vi "Main.vi"() -> ()   [LabVIEW 2019]
doc: "Self driving example made by ybbaek for ERP42."
uses:
  Ctrl/state.ctl
  <vilib>/userDefined/High Color/IMAQdx.ctl
  Ctrl/status.ctl
  Ctrl/system_hw.ctl
  Ctrl/joystick cfg.ctl
  Gmap/gmap_fgv-cmd.ctl
  Gmap/marker_info.ctl
  Ctrl/log_buffq.ctl
  Ctrl/error_modules.ctl
  Ctrl/agv_cmd_v.ctl
  Ctrl/cmd_common.ctl
  Ctrl/gps-databuf.ctl
  Ctrl/obstacle_info.ctl
  Ctrl/pid-in-params.ctl
  Ctrl/waypoint_buf.ctl
  Ctrl/pid-status.ctl
  Subvi/global_setting.vi
  Ctrl/pid-cfg.ctl
  Gmap/dll/GMap.NET.WindowsForms.dll
panel:
  out "State":T1
  out "Error Display":T3={"AGV"=0, "AGV Estop"=0, "Obstacle"=2, "Heading"=1, "Waypt"=2, "GNSS"=0, "VLP16"=0, "Cam"=0, "RPlidar"=0, "Joystic"=1}
  out "loop count out":T4
  out "Time info":T5={"Time_total"=2.602255344390869, "Time_run"=0.0, "Time_wait"=2.602255344390869} {"Time_total" format="%.1f"; "Time_run" format="%.1f"; "Time_wait" format="%.1f"}
  in  "ybbaek copyright":string="Made by ybbaek"
  in  "Tab_main":enum32{"Main UI", "Sub UI", "Config", "System"}(tab)
  out "point all":T6(graph)
  out "Image_color":T7(plugin-control)
  out "LiDAR Display":T8(graph)=[{"Array out"=[{"x"=0.0, "y"=0.0}, {"x"=0.7193398003386512, "y"=0.6946583704589973}, {"x"=0.0, "y"=0.0}, {"x"=-0.9271838545667873, "y"=0.37460659341591224}]}, {"Array out"=[{"x"=0.037211895365512664, "y"=0.3432387468560421}, {"x"=0.04793422512858862, "y"=0.3514966181363937}, {"x"=0.05832058142901035, "y"=0.36436205864741483}, {"x"=0.5627341150394717, "y"=3.0408693766373363}, {"x"=0.64680532100145, "y"=3.034839678916205}, {"x"=0.7366873283364822, "y"=3.05750172203851}, {"x"=0.8158698786760423, "y"=3.031635959522373}, {"x"=0.9331451610257764, "y"=3.131420821041812}, {"x"=0.004899685467144683, "y"=0.014968486307006838}, {"x"=1.049914434873501, "y"=2.9393674901148814}, {"x"=1.0224338842359812, "y"=1.9719484057312768}, {"x"=1.056603656991572, "y"=1.7959963180730734}, {"x"=1.0610931358520728, "y"=1.6950166428526934}, {"x"=1.0578713664954669, "y"=1.5944875107535377}, {"x"=1.0665021443408391, "y"=1.5125636312619686}, {"x"=1.077433024477614, "y"=1.4428578032034274}, {"x"=1.0850032011048054, "y"=1.3740064104989924}, {"x"=1.095072225331472, "y"=1.313035370356632}, {"x"=0.13957607278118947, "y"=0.14149234045339731}, {"x"=0.14291599956060283, "y"=0.13703655377158958}, {"x"=0.1465133078236048, "y"=0.1320659423567849}, {"x"=0.1386578275100177, "y"=0.09964722459859167}, {"x"=0.14122077174109132, "y"=0.09553503874940641}, {"x"=0.1444688686324124, "y"=0.09054830752736777}, {"x"=0.14738443732694032, "y"=0.08866694780932297}, {"x"=0.14995457808021992, "y"=0.08424740062923733}, {"x"=0.15169045746791707, "y"=0.08108023873407158}, {"x"=0.1550803380410649, "y"=0.07610946887916797}, {"x"=0.5644290746383124, "y"=0.24359265629927856}, {"x"=0.5639582150498643, "y"=0.2251748080442638}, {"x"=0.41414950492205704, "y"=0.14933268253404902}, {"x"=0.4146181630277808, "y"=0.13646988271215205}, {"x"=0.4184586846717039, "y"=0.12594176917459707}, {"x"=0.44769458462526207, "y"=0.12192439828522457}, {"x"=0.4515514564372801, "y"=0.10997201775620523}, {"x"=0.4606289556921582, "y"=0.0994863190491623}, {"x"=0.4600799668226086, "y"=0.08708895813194327}, {"x"=0.4048614011129938, "y"=0.06310553374168962}, {"x"=0.40636024710491037, "y"=0.05259669260358649}, {"x"=0.4111820157171695, "y"=0.04129058549797192}, {"x"=0.4536741901985323, "y"=0.03470920839929828}, {"x"=0.5839992182281244, "y"=0.000955567339076485}, {"x"=0.586069487141582, "y"=-0.014547121419821205}, {"x"=0.5882933358739553, "y"=-0.06150773094736755}, {"x"=0.5992636657008293, "y"=-0.0793933811523641}, {"x"=0.575868798189793, "y"=-0.09249697168796123}, {"x"=0.4794815805850259, "y"=-0.09211664550821055}, {"x"=0.5207405070619217, "y"=-0.1136588065434995}, {"x"=0.40395494215122685, "y"=-0.10247422706026608}, {"x"=0.37792320123187456, "y"=-0.10781026839152218}, {"x"=0.3495071946982059, "y"=-0.1103039929204306}, {"x"=0.3289166799304172, "y"=-0.11365657773992448}, {"x"=0.30733030791446936, "y"=-0.11672465179728503}, {"x"=0.3050947287304734, "y"=-0.1251090284546997}, {"x"=0.3038469355038735, "y"=-0.13379476740480148}, {"x"=0.30405676193652464, "y"=-0.27167912695066504}, {"x"=0.3099218476849613, "y"=-0.29154536238386586}, {"x"=0.3388604334873547, "y"=-0.33500127853004097}, {"x"=0.34325151630072614, "y"=-0.35700274376712055}, {"x"=0.3407582247030446, "y"=-0.37473468253849856}, {"x"=0.3258029246355666, "y"=-0.39787625814932875}, {"x"=0.3155139482560953, "y"=-0.40703310486476396}, {"x"=0.1343419152206783, "y"=-0.4670634323246042}, {"x"=0.11070702115716548, "y"=-0.43049297957865346}, {"x"=0.11046424140565235, "y"=-0.4761031546531421}, {"x"=0.09739123596280085, "y"=-0.4786932182072753}, {"x"=0.004218583737141675, "y"=-0.07688435179705115}, {"x"=0.05802099448158526, "y"=-0.4868045056276368}, {"x"=0.04608558674643472, "y"=-0.4956119260008145}, {"x"=0.01557949333511481, "y"=-0.7515885456068507}, {"x"=-0.0018576833489375396, "y"=-0.8514979735810151}, {"x"=-0.022647220319522755, "y"=-0.7616633793296085}, {"x"=-0.09417492708361101, "y"=-0.868659971225103}, {"x"=-0.11785941611955293, "y"=-0.8642506699632683}, {"x"=-0.14229004286206018, "y"=-0.8707000667292458}, {"x"=-0.1609050630122117, "y"=-0.841250147516799}, {"x"=-0.2067671415164568, "y"=-0.9523117132478806}, {"x"=-0.20605198625482285, "y"=-0.834178123340838}, {"x"=-0.2333515117149486, "y"=-0.847719077572487}, {"x"=-0.2594279084234967, "y"=-0.8518728839040539}, {"x"=-0.3389774409953587, "y"=-1.0251606493600105}, {"x"=-0.3728374985757233, "y"=-1.0348875299547278}, {"x"=-0.21982257555849657, "y"=-0.5453641309023074}, {"x"=-0.23306171365272346, "y"=-0.5352067825889877}, {"x"=-0.27818218393019845, "y"=-0.601266099612996}, {"x"=-0.2924118709245134, "y"=-0.5888985886741671}, {"x"=-0.30550719069246923, "y"=-0.5757112287728938}, {"x"=-0.285138558869652, "y"=-0.5004717796696813}, {"x"=-0.4124354308366926, "y"=-0.6129017685490489}, {"x"=-0.3722032482985255, "y"=-0.5194090314540422}, {"x"=-0.7050699279609969, "y"=-0.8482248503109743}, {"x"=-0.3534212598641885, "y"=-0.3929448600961842}, {"x"=-0.3687859639279288, "y"=-0.38861931926983306}, {"x"=-0.39927061762438265, "y"=-0.399052908649773}, {"x"=-0.7643321273706124, "y"=-0.6644237816101362}, {"x"=-0.767297911014162, "y"=-0.6311070953121213}, {"x"=-0.7686998824150671, "y"=-0.5985512119067692}, {"x"=-0.7271779246070609, "y"=-0.5341042299628113}, {"x"=-0.730511285151404, "y"=-0.5070688560407197}, {"x"=-0.7276478769936012, "y"=-0.47735063591316707}, {"x"=-0.7332296600619094, "y"=-0.45180286420683174}, {"x"=-0.7376706569933296, "y"=-0.4283118044264359}, {"x"=-0.7350246671034126, "y"=-0.4003844886474967}, {"x"=-0.7418987933431203, "y"=-0.37878117751021134}, {"x"=-0.7475662617627721, "y"=-0.35657081593147044}, {"x"=-0.5041435086062458, "y"=-0.21986205386601904}, {"x"=-0.48584433979299657, "y"=-0.19629385494993803}, {"x"=-0.4760784578208513, "y"=-0.1765201532373003}, {"x"=-0.4679334959572237, "y"=-0.15912669751255104}, {"x"=-0.46186928933121624, "y"=-0.14300003347089568}, {"x"=-0.4560366343728139, "y"=-0.12740815558635363}, {"x"=-0.4502754175244038, "y"=-0.1130491524657474}, {"x"=-0.4467093644643722, "y"=-0.09877749591803121}, {"x"=-0.44298273088963747, "y"=-0.08598175756263068}, {"x"=-0.4393424368145555, "y"=-0.07228959616603416}, {"x"=-0.4376169524302142, "y"=-0.06028652789547273}, {"x"=-0.43629870361981704, "y"=-0.048625520250862364}, {"x"=-0.43597758286292637, "y"=-0.036466385082705326}, {"x"=-0.4337740523176188, "y"=-0.025106205128448075}, {"x"=-0.43357219121954194, "y"=-0.012418433922397894}, {"x"=-0.4359989623973254, "y"=-0.0009512036877710461}, {"x"=-0.43962337625886316, "y"=0.010552229468602261}, {"x"=-0.4404266860988643, "y"=0.022479639053429236}, {"x"=-0.44495895343541736, "y"=0.0339203811543749}, {"x"=-0.45280773239569483, "y"=0.047092674405568156}, {"x"=-0.4578160839367756, "y"=0.06014562152638581}, {"x"=-0.46552826933189745, "y"=0.07321197274249847}, {"x"=-0.47641106321124965, "y"=0.08816319441766314}, {"x"=-0.4901086875913299, "y"=0.10389645974480644}, {"x"=-0.5103178534645616, "y"=0.12222213766467285}, {"x"=-0.5370139372294994, "y"=0.17400080810522456}, {"x"=-0.46408149329591586, "y"=0.1656228549453027}, {"x"=-0.4656495005595963, "y"=0.18005861581329152}, {"x"=-0.4663323638082487, "y"=0.19510093916998753}, {"x"=-0.46745010045348906, "y"=0.210111050604253}, {"x"=-0.4680972244411454, "y"=0.22531142552142344}, {"x"=-0.3747706718906415, "y"=0.1956131539304991}, {"x"=-0.36683941231682005, "y"=0.204521014986358}, {"x"=-0.3667965791811537, "y"=0.21713896932840876}, {"x"=-0.37017299397228004, "y"=0.23130975883779384}, {"x"=-0.318220561410615, "y"=0.21313065076500143}, {"x"=-0.3213045287871339, "y"=0.2276015427910756}, {"x"=-0.24212538367337458, "y"=0.227520023472707}, {"x"=-0.17947946669285567, "y"=0.18184435937264626}, {"x"=-0.16924099319043878, "y"=0.18298373896036188}, {"x"=-0.1677860822391545, "y"=0.1906930271584037}, {"x"=-0.16954711267984662, "y"=0.20105416330413897}, {"x"=-0.17052850865758717, "y"=0.2131877757635724}, {"x"=-0.17180789851886022, "y"=0.22645111725609354}, {"x"=-0.17303310157237145, "y"=0.24077332858986972}, {"x"=-0.1745382370945011, "y"=0.2558934666847587}, {"x"=-0.17570834500136337, "y"=0.27251539405487146}, {"x"=-0.148514703144379, "y"=0.24762864424362738}, {"x"=-0.13531890973055075, "y"=0.24055101884908958}, {"x"=-0.12622349307376365, "y"=0.23896169629515426}, {"x"=-0.11776445083836014, "y"=0.23962582106012587}, {"x"=-0.10315605611142512, "y"=0.2424687156883059}, {"x"=-0.09858183094858941, "y"=0.24867221920999485}, {"x"=-0.09247908731977739, "y"=0.2547324447503713}, {"x"=-0.0881002983385431, "y"=0.262352625168226}, {"x"=-0.0873557497448522, "y"=0.33892325530496537}, {"x"=-0.06613864879492504, "y"=0.32968127280083953}, {"x"=-0.06185317464036562, "y"=0.35134704678836914}, {"x"=-0.00018341309306920187, "y"=0.0012364706374559762}, {"x"=-0.042421581193537373, "y"=0.34943441365875816}, {"x"=-0.03273550342374527, "y"=0.3499723372148061}, {"x"=-0.024293544189698438, "y"=0.3501582837956332}, {"x"=-0.014938511138139295, "y"=0.3509321920043467}, {"x"=-0.004789280494373356, "y"=0.3512173476529117}, {"x"=0.0048920138106873946, "y"=0.35171598016137395}, {"x"=0.013560524982257915, "y"=0.352489254676232}, {"x"=0.02302380955838009, "y"=0.35274942125171443}, {"x"=0.03241116769680544, "y"=0.3434741856508718}, {"x"=0.04205573461848268, "y"=0.34721229483660243}, {"x"=0.051937519237767016, "y"=0.3554758171738643}, {"x"=0.68417575196985, "y"=3.054565206852931}, {"x"=0.7740347270876193, "y"=3.065281796387144}, {"x"=0.8538929235576769, "y"=3.0403668981059053}, {"x"=0.9711284589486772, "y"=3.1366035398532546}, {"x"=1.041383507715918, "y"=3.0678168870317686}, {"x"=1.0278480103439231, "y"=1.9318298398492655}, {"x"=1.040399634162634, "y"=1.8342287653764067}, {"x"=1.0503970797857973, "y"=1.7406191354737743}, {"x"=1.0601277685845496, "y"=1.655088929416164}, {"x"=1.062001244562704, "y"=1.5625040540898663}, {"x"=1.0700991338114112, "y"=1.4838996239018554}, {"x"=1.0845254893266352, "y"=1.420586859541092}, {"x"=1.0854238645260335, "y"=1.3448803280654271}, {"x"=1.0877327010534705, "y"=1.2763880957839278}, {"x"=0.14087035389941074, "y"=0.13949410701622764}, {"x"=0.14466196788817007, "y"=0.13482573028440104}, {"x"=0.14687291655966134, "y"=0.1316658987029624}, {"x"=0.14175064593549874, "y"=0.11887705572089544}, {"x"=0.2036264970682614, "y"=0.16841707808802925}, {"x"=0.13592407449410887, "y"=0.10000604218205987}, {"x"=0.14135771155859755, "y"=0.0975502941200914}, {"x"=0.14225736750876022, "y"=0.09443730136697859}, {"x"=0.1453994370555474, "y"=0.08904635705030223}, {"x"=0.14872128723328512, "y"=0.08640589519051754}, {"x"=0.1497717087020608, "y"=0.08147812757093183}, {"x"=0.1529452242949335, "y"=0.07813975214557874}, {"x"=0.15682442253056755, "y"=0.07537970879456893}, {"x"=0.5647472811675264, "y"=0.2540296654209641}, {"x"=0.5638885408067102, "y"=0.23591582407053377}, {"x"=0.5645154936678932, "y"=0.21828838702252315}, {"x"=0.4133143110507845, "y"=0.14420937133423556}, {"x"=0.4152953038207189, "y"=0.1319388992089019}, {"x"=0.42070181991580574, "y"=0.12187689986018242}, {"x"=0.41019463382308746, "y"=0.10632226898793665}, {"x"=0.4607697813923746, "y"=0.10796652747784073}, {"x"=0.4595728307656681, "y"=0.09480704468566964}, {"x"=0.4615395686039659, "y"=0.08190109347783492}, {"x"=0.4039610364961172, "y"=0.05902155108926479}, {"x"=0.4078632344447768, "y"=0.04861218456565249}, {"x"=0.4148145551337871, "y"=0.03743173585553142}, {"x"=0.4555144394149477, "y"=0.029980751899943522}, {"x"=0.4454442737995556, "y"=-0.007046200336816244}, {"x"=0.40558405794575164, "y"=-0.01837313093234705}, {"x"=0.5870349933318487, "y"=-0.06834410438272143}, {"x"=0.5825244442519296, "y"=-0.0836511915574467}, {"x"=0.4929294557879973, "y"=-0.10014764908148785}, {"x"=0.4196071385781955, "y"=-0.09844211118326883}, {"x"=0.3942699940919931, "y"=-0.10495318841607298}, {"x"=0.36809742892892505, "y"=-0.109363077937277}, {"x"=0.3385160682701253, "y"=-0.11019469825239267}, {"x"=0.3182903986529594, "y"=-0.11447394736506725}, {"x"=0.3032784647494663, "y"=-0.11889169575376882}, {"x"=0.3049481648503731, "y"=-0.12807099302492214}, {"x"=0.3046065295002057, "y"=-0.13761513247401344}, {"x"=0.3043912180306484, "y"=-0.2637300682247252}, {"x"=0.3054171367735939, "y"=-0.27986324350478725}, {"x"=0.31311274043158194, "y"=-0.30088781012102306}, {"x"=0.3523944987568351, "y"=-0.3547084961569415}, {"x"=0.3415368298179463, "y"=-0.3634613547241401}, {"x"=0.3524178717309416, "y"=-0.39485086575140443}, {"x"=0.31908555382111603, "y"=-0.39913081733019773}, {"x"=0.12997044339241726, "y"=-0.47115204164301194}, {"x"=0.10505526757844699, "y"=-0.42881889038849597}, {"x"=0.1046592082535379, "y"=-0.4763890349575047}, {"x"=0.06527164362595625, "y"=-0.4805877781824733}, {"x"=0.05278646127519131, "y"=-0.48689696241201047}, {"x"=0.3386987778362214, "y"=-3.274027395714985}, {"x"=0.025957529292859365, "y"=-0.7207827475550524}, {"x"=0.01162380532798078, "y"=-0.8524207512430099}, {"x"=-0.011422689634622552, "y"=-0.8376721224091865}, {"x"=-0.08307037095562, "y"=-0.898668772946571}, {"x"=-0.10411225420149112, "y"=-0.8634962078811257}, {"x"=-0.12842874128580306, "y"=-0.8690617402761119}, {"x"=-0.14986750133717497, "y"=-0.8595324205886313}, {"x"=-0.17043851785727526, "y"=-0.8365642677825866}, {"x"=-0.2150687033246629, "y"=-0.9373945355880031}, {"x"=-0.21778331896159028, "y"=-0.8373935684503878}, {"x"=-0.24578382552810385, "y"=-0.8553889823400642}, {"x"=-0.28307706457464193, "y"=-0.8961012431705494}, {"x"=-0.35544480560474834, "y"=-1.034118581289691}, {"x"=-0.2141042776522463, "y"=-0.5559473183594016}, {"x"=-0.22620957901224753, "y"=-0.5419333804658113}, {"x"=-0.24236435690757, "y"=-0.5403883612743524}, {"x"=-0.28505726329887, "y"=-0.5955438011939664}, {"x"=-0.29777273816175426, "y"=-0.5828392972403725}, {"x"=-0.31132675134567095, "y"=-0.5711618893943736}, {"x"=-0.29361851874449085, "y"=-0.5022163158941484}, {"x"=-0.418055248346186, "y"=-0.6054402297751684}, {"x"=-0.7024675187103798, "y"=-0.8713552362021372}, {"x"=-0.3493476679235393, "y"=-0.3992323345075954}, {"x"=-0.3598912709755358, "y"=-0.3897544394559393}, {"x"=-0.3784374459844478, "y"=-0.3897507690521831}, {"x"=-0.41910536477373445, "y"=-0.41028397874871375}, {"x"=-0.7630706703020157, "y"=-0.6467017972951926}, {"x"=-0.7653163194517437, "y"=-0.614917875558059}, {"x"=-0.771485862982975, "y"=-0.5863195060864123}, {"x"=-0.7256074092092951, "y"=-0.5196634850560259}, {"x"=-0.7225359964678987, "y"=-0.48907870921574637}, {"x"=-0.7316420792426782, "y"=-0.46610741024087005}, {"x"=-0.7351413730499343, "y"=-0.4414446869430613}, {"x"=-0.7371148283931629, "y"=-0.4151839709850541}, {"x"=-0.733924960023978, "y"=-0.3886957718496593}, {"x"=-0.743501136253052, "y"=-0.36892554857372045}, {"x"=-0.5212418238111429, "y"=-0.23617159780556485}, {"x"=-0.4960873673387058, "y"=-0.20818579194304304}, {"x"=-0.48117061967940855, "y"=-0.18636210654887417}, {"x"=-0.47138059339341626, "y"=-0.168227780619227}, {"x"=-0.46513920483608606, "y"=-0.1516940428113563}, {"x"=-0.4590349480681474, "y"=-0.13597234627700297}, {"x"=-0.45373331656080873, "y"=-0.12064960606122574}, {"x"=-0.4479402014885775, "y"=-0.10573380911691682}, {"x"=-0.44457945085334866, "y"=-0.09323183136104837}, {"x"=-0.4406259337607172, "y"=-0.07955406336257143}, {"x"=-0.438200982952092, "y"=-0.06671177587068398}, {"x"=-0.4366171481572478, "y"=-0.05445609180828143}, {"x"=-0.4354166419328846, "y"=-0.04264502231081791}, {"x"=-0.4339237471993289, "y"=-0.030580739305859018}, {"x"=-0.4335765385183767, "y"=-0.019167296273147325}, {"x"=-0.4336899858120299, "y"=-0.0072151719564631945}, {"x"=-0.43822888027642554, "y"=0.004302440199505958}, {"x"=-0.43970624941831693, "y"=0.016075267415408327}, {"x"=-0.44215144199202855, "y"=0.027406246448023953}, {"x"=-0.4482228403567289, "y"=0.039953540300533656}, {"x"=-0.45564325347687923, "y"=0.053299043715665406}, {"x"=-0.46126829400407676, "y"=0.06623866655186098}, {"x"=-0.4697270563321256, "y"=0.0800546222872615}, {"x"=-0.4827653473306562, "y"=0.0961648684120708}, {"x"=-0.49943682417100876, "y"=0.11272470298021144}, {"x"=-0.5273462266081955, "y"=0.13255195125722483}, {"x"=-0.5907054678168859, "y"=0.1638171245359714}, {"x"=-0.5561032586373484, "y"=0.17167750502882528}, {"x"=-0.4638415561984629, "y"=0.17284678401228107}, {"x"=-0.46528947420424066, "y"=0.18710412928297776}, {"x"=-0.46758216578865297, "y"=0.20300734158249711}, {"x"=-0.4675470533001976, "y"=0.21771039352842617}, {"x"=-0.46980834082055095, "y"=0.2348780223763838}, {"x"=-0.3716843976287295, "y"=0.2008904143043377}, {"x"=-0.36512371869559074, "y"=0.20908188000375139}, {"x"=-0.361088043164779, "y"=0.2203279943253483}, {"x"=-0.3366952424332568, "y"=0.2182610277232525}, {"x"=-0.320284358249612, "y"=0.22076895130573543}, {"x"=-0.3241672532540743, "y"=0.23646808329605257}, {"x"=-0.1813842335345227, "y"=0.18029925769423935}, {"x"=-0.17445776505200078, "y"=0.1825396894186601}, {"x"=-0.16770514735426642, "y"=0.18473016416082078}, {"x"=-0.16852708540716116, "y"=0.1963420076910884}, {"x"=-0.16928188551480808, "y"=0.20776824405224062}, {"x"=-0.170922566662934, "y"=0.219881163825724}, {"x"=-0.1721789491288038, "y"=0.23428609002008804}, {"x"=-0.17346253854849844, "y"=0.24873944242984602}, {"x"=-0.17501652116040026, "y"=0.26520610818929335}, {"x"=-0.17657379175860174, "y"=0.28292038820839677}, {"x"=-0.14104420185130634, "y"=0.24245985878930137}, {"x"=-0.13009106473664403, "y"=0.23944219526993626}, {"x"=-0.12093484089413561, "y"=0.23944274212828023}, {"x"=-0.11358132542809246, "y"=0.23997819174666218}, {"x"=-0.10529675589785026, "y"=0.24072838573252747}, {"x"=-0.10043881698271782, "y"=0.24684872704373445}, {"x"=-0.09473578958399388, "y"=0.2514988919894027}, {"x"=-0.09011184118675057, "y"=0.2584935561632704}, {"x"=-0.08575197566726976, "y"=0.2686458610683589}, {"x"=-0.07276691295892505, "y"=0.3364714532890245}]}, {"Array out"=[{"x"=0.037211895365512664, "y"=0.3432387468560421}, {"x"=0.04793422512858862, "y"=0.3514966181363937}, {"x"=0.05832058142901035, "y"=0.36436205864741483}, {"x"=0.004899685467144683, "y"=0.014968486307006838}, {"x"=0.13957607278118947, "y"=0.14149234045339731}, {"x"=-0.4663323638082487, "y"=0.19510093916998753}, {"x"=-0.46745010045348906, "y"=0.210111050604253}, {"x"=-0.4680972244411454, "y"=0.22531142552142344}, {"x"=-0.3747706718906415, "y"=0.1956131539304991}, {"x"=-0.36683941231682005, "y"=0.204521014986358}, {"x"=-0.3667965791811537, "y"=0.21713896932840876}, {"x"=-0.37017299397228004, "y"=0.23130975883779384}, {"x"=-0.318220561410615, "y"=0.21313065076500143}, {"x"=-0.3213045287871339, "y"=0.2276015427910756}, {"x"=-0.24212538367337458, "y"=0.227520023472707}, {"x"=-0.17947946669285567, "y"=0.18184435937264626}, {"x"=-0.16924099319043878, "y"=0.18298373896036188}, {"x"=-0.1677860822391545, "y"=0.1906930271584037}, {"x"=-0.16954711267984662, "y"=0.20105416330413897}, {"x"=-0.17052850865758717, "y"=0.2131877757635724}, {"x"=-0.17180789851886022, "y"=0.22645111725609354}, {"x"=-0.17303310157237145, "y"=0.24077332858986972}, {"x"=-0.1745382370945011, "y"=0.2558934666847587}, {"x"=-0.17570834500136337, "y"=0.27251539405487146}, {"x"=-0.148514703144379, "y"=0.24762864424362738}, {"x"=-0.13531890973055075, "y"=0.24055101884908958}, {"x"=-0.12622349307376365, "y"=0.23896169629515426}, {"x"=-0.11776445083836014, "y"=0.23962582106012587}, {"x"=-0.10315605611142512, "y"=0.2424687156883059}, {"x"=-0.09858183094858941, "y"=0.24867221920999485}, {"x"=-0.09247908731977739, "y"=0.2547324447503713}, {"x"=-0.0881002983385431, "y"=0.262352625168226}, {"x"=-0.0873557497448522, "y"=0.33892325530496537}, {"x"=-0.06613864879492504, "y"=0.32968127280083953}, {"x"=-0.06185317464036562, "y"=0.35134704678836914}, {"x"=-0.00018341309306920187, "y"=0.0012364706374559762}, {"x"=-0.042421581193537373, "y"=0.34943441365875816}, {"x"=-0.03273550342374527, "y"=0.3499723372148061}, {"x"=-0.024293544189698438, "y"=0.3501582837956332}, {"x"=-0.014938511138139295, "y"=0.3509321920043467}, {"x"=-0.004789280494373356, "y"=0.3512173476529117}, {"x"=0.0048920138106873946, "y"=0.35171598016137395}, {"x"=0.013560524982257915, "y"=0.352489254676232}, {"x"=0.02302380955838009, "y"=0.35274942125171443}, {"x"=0.03241116769680544, "y"=0.3434741856508718}, {"x"=0.04205573461848268, "y"=0.34721229483660243}, {"x"=0.051937519237767016, "y"=0.3554758171738643}, {"x"=0.14087035389941074, "y"=0.13949410701622764}, {"x"=-0.46758216578865297, "y"=0.20300734158249711}, {"x"=-0.4675470533001976, "y"=0.21771039352842617}, {"x"=-0.46980834082055095, "y"=0.2348780223763838}, {"x"=-0.3716843976287295, "y"=0.2008904143043377}, {"x"=-0.36512371869559074, "y"=0.20908188000375139}, {"x"=-0.361088043164779, "y"=0.2203279943253483}, {"x"=-0.3366952424332568, "y"=0.2182610277232525}, {"x"=-0.320284358249612, "y"=0.22076895130573543}, {"x"=-0.3241672532540743, "y"=0.23646808329605257}, {"x"=-0.1813842335345227, "y"=0.18029925769423935}, {"x"=-0.17445776505200078, "y"=0.1825396894186601}, {"x"=-0.16770514735426642, "y"=0.18473016416082078}, {"x"=-0.16852708540716116, "y"=0.1963420076910884}, {"x"=-0.16928188551480808, "y"=0.20776824405224062}, {"x"=-0.170922566662934, "y"=0.219881163825724}, {"x"=-0.1721789491288038, "y"=0.23428609002008804}, {"x"=-0.17346253854849844, "y"=0.24873944242984602}, {"x"=-0.17501652116040026, "y"=0.26520610818929335}, {"x"=-0.17657379175860174, "y"=0.28292038820839677}, {"x"=-0.14104420185130634, "y"=0.24245985878930137}, {"x"=-0.13009106473664403, "y"=0.23944219526993626}, {"x"=-0.12093484089413561, "y"=0.23944274212828023}, {"x"=-0.11358132542809246, "y"=0.23997819174666218}, {"x"=-0.10529675589785026, "y"=0.24072838573252747}, {"x"=-0.10043881698271782, "y"=0.24684872704373445}, {"x"=-0.09473578958399388, "y"=0.2514988919894027}, {"x"=-0.09011184118675057, "y"=0.2584935561632704}, {"x"=-0.08575197566726976, "y"=0.2686458610683589}, {"x"=-0.07276691295892505, "y"=0.3364714532890245}]}, {"Array out"=[]}, {"Array out"=[]}]
  in  "Tab sub":enum32{"Set ", "Info", "Map waypoint"}(tab)=enum."Info"
  in  "Speed":u16(slide)=33 scale=0.0..100.0
  in  "set state value":T1
  in  "state change":bool
  in  "full scale":bool=TRUE
  in  "ratio":dbl=10.0 format="%#_13g"
  in  "Scale_map":dbl(slide)=5.0 min=0.0 scale=5.0..100.0
  out "process_all":u8(slide) scale=0.0..100.0
  out "process_curr":dbl(slide)=nan scale=0.0..1.0
  out "stop time":dbl(slide)=2.7272372245788574 scale=0.0..5.0
  out "Pid dt":u32=100
  out "Heading":dbl
  out "Speed_control_PID":T9(graph)={"output high"=40.0, "output low"=15.0, "output"=0.0}
  out "Distance_left":dbl format="%.1f"
  out "D_gap":dbl format="%.1f"
  out "Map_Total":T10(graph)=[{"stop pt array out"=[]}, {"stop pt array out"=[]}, {"stop pt array out"=[{"X"=4530998.623923, "Y"=6178450.805513}, {"X"=4530998.538097, "Y"=6178450.804328}, {"X"=4530998.436351, "Y"=6178450.81696}, {"X"=4530998.335494, "Y"=6178450.839631}, {"X"=4530998.287734, "Y"=6178450.881083}, {"X"=4530998.369203, "Y"=6178451.026592}, {"X"=4530998.616099, "Y"=6178451.104199}, {"X"=4530998.899282, "Y"=6178451.204366}, {"X"=4530999.432829, "Y"=6178451.227778}, {"X"=4530999.994657, "Y"=6178451.1834}, {"X"=4531000.491916, "Y"=6178451.184252}, {"X"=4531000.925496, "Y"=6178451.240374}, {"X"=4531001.380332, "Y"=6178451.342912}, {"X"=4531001.869676, "Y"=6178451.447932}, {"X"=4531002.371383, "Y"=6178451.498979}, {"X"=4531002.905819, "Y"=6178451.53243}, {"X"=4531003.356208, "Y"=6178451.584774}, {"X"=4531003.754389, "Y"=6178451.628375}, {"X"=4531004.172048, "Y"=6178451.698315}, {"X"=4531004.577345, "Y"=6178451.822228}, {"X"=4531004.966722, "Y"=6178451.959958}, {"X"=4531005.304781, "Y"=6178452.098985}, {"X"=4531005.558793, "Y"=6178452.256904}, {"X"=4531005.663298, "Y"=6178452.468907}, {"X"=4531005.735073, "Y"=6178452.698506}, {"X"=4531005.808628, "Y"=6178452.948183}, {"X"=4531005.871598, "Y"=6178453.271912}, {"X"=4531005.874357, "Y"=6178453.496547}, {"X"=4531005.809877, "Y"=6178453.736296}, {"X"=4531005.695859, "Y"=6178453.997419}, {"X"=4531005.514602, "Y"=6178454.273656}, {"X"=4531005.263439, "Y"=6178454.53489}, {"X"=4531004.89372, "Y"=6178454.812535}, {"X"=4531004.439065, "Y"=6178455.099032}, {"X"=4531003.810977, "Y"=6178455.363081}, {"X"=4531003.261601, "Y"=6178455.548003}, {"X"=4531002.709556, "Y"=6178455.702809}, {"X"=4531002.017699, "Y"=6178455.827609}, {"X"=4531001.45765, "Y"=6178455.892064}, {"X"=4531000.845393, "Y"=6178455.947777}, {"X"=4531000.166788, "Y"=6178456.028643}, {"X"=4530999.390883, "Y"=6178456.172335}, {"X"=4530998.64593, "Y"=6178456.278353}, {"X"=4530997.881499, "Y"=6178456.358033}, {"X"=4530997.114399, "Y"=6178456.407596}, {"X"=4530996.505611, "Y"=6178456.308947}, {"X"=4530996.309053, "Y"=6178456.025486}, {"X"=4530996.530954, "Y"=6178455.627487}, {"X"=4530996.701536, "Y"=6178455.230783}, {"X"=4530996.904848, "Y"=6178454.816484}, {"X"=4530997.126748, "Y"=6178454.418484}, {"X"=4530997.382268, "Y"=6178454.012928}, {"X"=4530997.604168, "Y"=6178453.614928}, {"X"=4530997.677451, "Y"=6178453.281051}, {"X"=4530997.953338, "Y"=6178452.911871}, {"X"=4530998.350449, "Y"=6178452.556397}, {"X"=4530998.886482, "Y"=6178452.22089}, {"X"=4530999.254422, "Y"=6178451.923168}, {"X"=4530999.465739, "Y"=6178451.599218}, {"X"=4530999.52666, "Y"=6178451.319314}, {"X"=4530999.555832, "Y"=6178451.261562}, {"X"=4530999.57442, "Y"=6178451.277862}, {"X"=4530999.57531, "Y"=6178451.287901}, {"X"=4530999.561169, "Y"=6178451.321796}, {"X"=4530999.562948, "Y"=6178451.341874}, {"X"=4530999.582425, "Y"=6178451.368212}, {"X"=4530999.584204, "Y"=6178451.38829}, {"X"=4530999.552364, "Y"=6178451.415925}, {"X"=4530999.520524, "Y"=6178451.44356}]}]
  out "joystick":cluster{"X":dbl, "Y":dbl}[](graph)
  out "Map_Current":T11(graph)=[{"heading_curr "=[]}, {"heading_curr "=[]}, {"heading_curr "=[{"x"=0.0, "y"=0.0}, {"x"=0.0, "y"=0.0}, {"x"=0.0, "y"=0.0}, {"x"=0.0, "y"=0.0}, {"x"=0.0, "y"=0.0}, {"x"=0.0, "y"=0.0}]}, {"heading_curr "=[]}, {"heading_curr "=[{"x"=0.0, "y"=0.0}, {"x"=0.0, "y"=0.0}]}, {"heading_curr "=[{"x"=0.0, "y"=0.0}, {"x"=0.0, "y"=0.0}]}, {"heading_curr "=[{"x"=0.0, "y"=0.0}, {"x"=3.6739403974420594e-16, "y"=6.0}]}, {"heading_curr "=[{"x"=0.0, "y"=0.0}, {"x"=3.6739403974420594e-16, "y"=6.0}]}]
  in  "zoom-center":bool
  in  "GMapControl":refnum<k24>(container)
  out "Lat":dbl format="%.16f"
  out "Lon":dbl format="%.16f"
  out "Lat_DbClk":dbl format="%.16f"
  out "Lon_DbClk":dbl format="%.16f"
  in  "zoom":dbl(slide) scale=3.0..20.0
  in  "PinDropMrkr":T12(ring)=enum."red_dot" caption="Pin Drop Marker"
  in  "SetMapProvider":u16(ring)=17 items=["None", "OpenStreetMap", "OpenStreet4UMap", "OpenCycleMap", "OpenCycleLandscapeMap", "OpenCycleTransportMap", "OpenStreetMapQuest", "OpenStreetMapQuestSattelite", "OpenStreetMapQuestHybrid", "OpenSeaMapHybrid", "WikiMapiaMap", "BingMap", "BingSatelliteMap", "BingHybridMap", "YahooMap", "YahooSatelliteMap", "YahooHybridMap", "GoogleMap", "GoogleSatelliteMap", "GoogleHybridMap", "GoogleTerrainMap", "GoogleChinaMap", "GoogleChinaSatelliteMap", "GoogleChinaHybridMap", "GoogleChinaTerrainMap", "GoogleKoreaMap", "GoogleKoreaSatelliteMap", "GoogleKoreaHybridMap", "NearMap", "NearSatelliteMap", "NearHybridMap", "OviMap", "OviSatelliteMap", "OviHybridMap", "OviTerrainMap", "YandexMap", "YandexSatelliteMap", "YandexHybridMap", "LithuaniaMap", "Lithuania 2.5d Map", "LithuaniaOrtoFotoMap", "LithuaniaOrtoFotoMapOld", "LithuaniaHybridMap", "LithuaniaHybridMapOld", "LithuaniaTOP50", "LatviaMap", "MapBender, WMS demo", "TurkeyMap", "CloudMade, Demo", "SpainMap", "CzechMap", "CzechSatelliteMap", "CzechHybridMap", "CzechTuristMap", "CzechHistoryMap", "ArcGIS_Imagery_World_2D_Map", "ArcGIS_ShadedRelief_World_2D_Map", "ArcGIS_StreetMap_World_2D_Map", "ArcGIS_Topo_US_2D_Map", "ArcGIS_World_Physical_Map", "ArcGIS_World_Shaded_Relief_Map", "ArcGIS_World_Street_Map", "ArcGIS_World_Terrain_Base_Map", "ArcGIS_World_Topo_Map", "ArcGIS_DarbAE_Q2_2011_NAVTQ_Eng_V5_MapProvider"]
  out "latlong out":cluster{dbl, dbl}={530126.7583503594, 175270.68061157822} {"?" format="%.8f"; "?" format="%.8f"}
  in  "Tap_config":T13(tab)=enum."Vision"
  in  "AGV-2":enum32{"Status", "Common"}(tab)
  out "batt":dbl(slide) scale=26.0..29.0
  out "AGV velocity Chart":T14(graph)
  out "System Feedback":T15
  in  "AGV cfg":T16={"Port"="COM6", "speed limits"={"speed-limit"=0.0, "steer-limit"=0.0}, "limits"={"speed limits"={"max"=100.0, "min"=0.0}, "steer limits"={"max"=500.0, "min"=0.0}}}
  in  "Lookahead cfg":T17={"lookahead points"=64.0, "lookahead distance"=2.0} {"lookahead distance" format="%.1f"; "lookahead points" format="%#_13g"}
  in  "State machine cfg":T18
  out "Slide":cluster{dbl, dbl, dbl}(slide) scale=0.0..1.0
  out "Stop point count":u32(slide)
  in  "Tab_Lidar-config":enum32{"VLP16", "Tim571", "RPLiar A123"}(tab)
  in  "TIM571 cfg":T19 {"h range" scale=-180.0..180.0}
  in  "RPLidar cfg":T20={"port"="COM3", "dt"=4, "cicle"=28, "speed"=500, "rate"=115200} {"speed" scale=100.0..1000.0}
  out "LiDAR Display for cfg":T8(graph)=[{"Array out"=[{"x"=0.0, "y"=0.0}, {"x"=0.7193398003386512, "y"=0.6946583704589973}, {"x"=0.0, "y"=0.0}, {"x"=-0.9271838545667873, "y"=0.37460659341591224}]}, {"Array out"=[]}, {"Array out"=[]}, {"Array out"=[]}, {"Array out"=[]}]
  in  "lidat setting tab":enum32{"Range", "Limit", "Graph"}(tab)
  in  "VLP16 cfg":T21={"h range"={46, -68}, "v range"={8, -4}} {"v range" scale=-15.0..15.0; "h range" scale=-180.0..180.0}
  in  "Obstacle limit cfg":cluster{"Range":dbl, "Points":u16}={"Range"=1.0, "Points"=110} {"Points" min=10 max=5000 scale=10.0..100.0; "Range" min=0.5 max=200.0 scale=0.5..20.0}
  in  "Lidar graph scale":dbl(slide)=1.0 min=1.0 scale=1.0..10.0
  in  "decrease ratio":dbl(slide)=1.1 min=1.0 max=2.0 scale=1.0..2.0
  in  "PID cfg":T22={"PID gains"={"proportional gain (Kc)"=0.01, "integral time (Ti, min)"=0.0, "derivative time (Td, min)"=0.0}, "PID limits"={"output high"=40.0, "output low"=15.0}, "dt_pid"=100} {"PID limits"."output low" format="%.3f"; "PID limits"."output high" format="%.3f"; "PID gains"."derivative time (Td, min)" format="%.4f"; "PID gains"."integral time (Ti, min)" format="%.4f"; "PID gains"."proportional gain (Kc)" format="%.4f"}
  out "Speed_control_PID 2":T9(graph)={"output high"=40.0, "output low"=15.0, "output"=0.0}
  out "Image_binary 2":T7(plugin-control)
  in  "speed-steer_global":cluster{"speed":dbl, "steer":dbl} {"speed" scale=0.0..200.0; "steer" scale=8.0..40.0}
  in  "Record waypoint":bool
  in  "GPS cfg":T23={"Port"="COM10", "PwrPak7_heading select"="", "PwrPak7_mode select"=[]}
  out "Image_binary":T7(plugin-control)
  out "Image_gray":T7(plugin-control)
  in  "Tab vision-setting":enum32{"Port ", "Config", "camera attrib"}(tab)
  in  "camera cfg":cluster{"Port":T24, "Camera file":path}={"Port"="cam1", "Camera file"=path "C:/AGV/Config/camera/MS_LifeCam_30fps_160x120.icd"}
  in  "Vison cfg":T25 {"Threshold Range"."Upper value" scale=0.0..255.0; "Threshold Range"."Lower value" scale=0.0..255.0}
  in  "camera_attrib":cluster{"brightness":u16, "ExposureTimeAbs":dbl}={"brightness"=0, "ExposureTimeAbs"=15000.0} {"brightness" scale=0.0..10.0; "ExposureTimeAbs" scale=0.0..30000.0}
  in  "config save":bool
  in  "config load":bool
  in  "config_file-name":string="user1"
  in  "waypoint files cfg":T26={"Waypoint array"=[{"sel"=TRUE, "inv"=FALSE, "path"=path "C:/AGV/Config/waypoint/wpt_shinsung-circle_20201004-1.txt"}]}
  out "Total map cfg":T27(graph)=[{"ref waypt 0703 A \ngoal point start"=[]}, {"ref waypt 0703 A \ngoal point start"=[{"X"=4530998.623923, "Y"=6178450.805513}, {"X"=4530998.538097, "Y"=6178450.804328}, {"X"=4530998.436351, "Y"=6178450.81696}, {"X"=4530998.335494, "Y"=6178450.839631}, {"X"=4530998.287734, "Y"=6178450.881083}, {"X"=4530998.369203, "Y"=6178451.026592}, {"X"=4530998.616099, "Y"=6178451.104199}, {"X"=4530998.899282, "Y"=6178451.204366}, {"X"=4530999.432829, "Y"=6178451.227778}, {"X"=4530999.994657, "Y"=6178451.1834}, {"X"=4531000.491916, "Y"=6178451.184252}, {"X"=4531000.925496, "Y"=6178451.240374}, {"X"=4531001.380332, "Y"=6178451.342912}, {"X"=4531001.869676, "Y"=6178451.447932}, {"X"=4531002.371383, "Y"=6178451.498979}, {"X"=4531002.905819, "Y"=6178451.53243}, {"X"=4531003.356208, "Y"=6178451.584774}, {"X"=4531003.754389, "Y"=6178451.628375}, {"X"=4531004.172048, "Y"=6178451.698315}, {"X"=4531004.577345, "Y"=6178451.822228}, {"X"=4531004.966722, "Y"=6178451.959958}, {"X"=4531005.304781, "Y"=6178452.098985}, {"X"=4531005.558793, "Y"=6178452.256904}, {"X"=4531005.663298, "Y"=6178452.468907}, {"X"=4531005.735073, "Y"=6178452.698506}, {"X"=4531005.808628, "Y"=6178452.948183}, {"X"=4531005.871598, "Y"=6178453.271912}, {"X"=4531005.874357, "Y"=6178453.496547}, {"X"=4531005.809877, "Y"=6178453.736296}, {"X"=4531005.695859, "Y"=6178453.997419}, {"X"=4531005.514602, "Y"=6178454.273656}, {"X"=4531005.263439, "Y"=6178454.53489}, {"X"=4531004.89372, "Y"=6178454.812535}, {"X"=4531004.439065, "Y"=6178455.099032}, {"X"=4531003.810977, "Y"=6178455.363081}, {"X"=4531003.261601, "Y"=6178455.548003}, {"X"=4531002.709556, "Y"=6178455.702809}, {"X"=4531002.017699, "Y"=6178455.827609}, {"X"=4531001.45765, "Y"=6178455.892064}, {"X"=4531000.845393, "Y"=6178455.947777}, {"X"=4531000.166788, "Y"=6178456.028643}, {"X"=4530999.390883, "Y"=6178456.172335}, {"X"=4530998.64593, "Y"=6178456.278353}, {"X"=4530997.881499, "Y"=6178456.358033}, {"X"=4530997.114399, "Y"=6178456.407596}, {"X"=4530996.505611, "Y"=6178456.308947}, {"X"=4530996.309053, "Y"=6178456.025486}, {"X"=4530996.530954, "Y"=6178455.627487}, {"X"=4530996.701536, "Y"=6178455.230783}, {"X"=4530996.904848, "Y"=6178454.816484}, {"X"=4530997.126748, "Y"=6178454.418484}, {"X"=4530997.382268, "Y"=6178454.012928}, {"X"=4530997.604168, "Y"=6178453.614928}, {"X"=4530997.677451, "Y"=6178453.281051}, {"X"=4530997.953338, "Y"=6178452.911871}, {"X"=4530998.350449, "Y"=6178452.556397}, {"X"=4530998.886482, "Y"=6178452.22089}, {"X"=4530999.254422, "Y"=6178451.923168}, {"X"=4530999.465739, "Y"=6178451.599218}, {"X"=4530999.52666, "Y"=6178451.319314}, {"X"=4530999.555832, "Y"=6178451.261562}, {"X"=4530999.57442, "Y"=6178451.277862}, {"X"=4530999.57531, "Y"=6178451.287901}, {"X"=4530999.561169, "Y"=6178451.321796}, {"X"=4530999.562948, "Y"=6178451.341874}, {"X"=4530999.582425, "Y"=6178451.368212}, {"X"=4530999.584204, "Y"=6178451.38829}, {"X"=4530999.552364, "Y"=6178451.415925}, {"X"=4530999.520524, "Y"=6178451.44356}]}]
  in  "test waypoint":bool
  in  "stop points edit":bool
  in  "stop point config":cluster{"distance":dbl, "time":dbl}={"distance"=1.0, "time"=5.0}
  in  "Joystick cfg":T28={"Type"=enum."Logitech F710", "steer limit"={"min"=10.0, "max"=42.0, "scale"=0.0, "offset"=0.0}, "speed limit"={"min"=10.0, "max"=42.0, "pwm max"=0.0}, "ID"=0, "joystick max"=0.0}
  out "LiDAR img":T7(plugin-control)
  in  "Joystick\ncontrol":bool
  in  "HW info":T29={"AGV"=enum."Ycar", "Lidar 1"=enum."RPLidar A2", "Lidar 2"=enum."none", "GPS"=enum."none", "Camera"=enum."MS LifeCam", "Joystick"=enum."joystick"}
  in  "Steer":i16(slide) scale=-2000.0..2000.0
  in  "use event":bool
  in  "pause-resume":bool
  in  "Checking":bool
  in  "start-stop":bool
  in  "close":bool
  in  "System status":string="\r\n00:38:31.5 - System start \r\n00:38:31.5 - UDP start \r\n00:38:31.6 - Logging loop finish \r\n00:38:31.6 - Jostick fail ### \r\n00:38:31.6 - UDP finish \r\n00:38:35.1 - VLP16 loop finish \r\n00:38:35.2 - F9P loop finish \r\n00:38:35.2 - Camera loop finish \r\n00:38:35.2 - Scout finish \r\n00:38:35.2 - Tim571 hw finish \r\n00:38:35.2 - RPLidar loop finish \r\n00:38:35.2 - GPS  finish \r\n00:38:35.2 - Producer fihish \r\n00:38:35.3 - Vision loop finish \r\n00:38:35.3 - Display Lidar finish \r\n00:38:35.3 - Timer loop finish \r\n00:38:35.5 - TCP loop finish \r\n00:38:36.5 - State loop finish \r\n00:38:36.6 - Shut down "
  # "System status"
  # "Set-Info"
  # "Process"
  # "<Xbox>\njoy max: 32767\nsteer min 10 / scale 16\nsteer max 42 / offset 26\nspeed min 10 / pwm max 255\nspeed max 200"
  # "AGV"
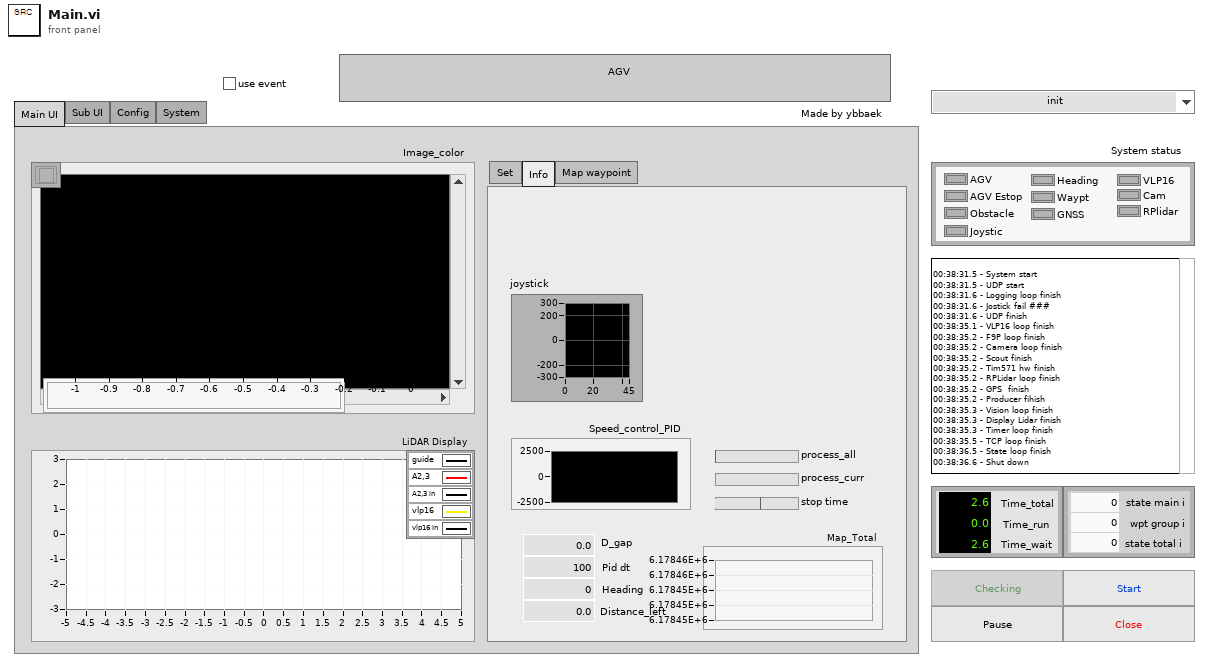
[diagram p1: front panel]
types:
  T1 = typedef "state.ctl" = enum16{"init", "Test circular track", "start point", "start heading adjust", "wait before start", "stop point check", "stop point start", "end point", "entering ending point", "move", "move heading adjust"}
  T2 = typedef "status.ctl" = u16
  T3 = cluster{"AGV":T2, "AGV Estop":T2, "Obstacle":T2, "Heading":T2, "Waypt":T2, "GNSS":T2, "VLP16":T2, "Cam":T2, "RPlidar":T2, "Joystic":T2}
  T4 = cluster{"wpt group i":i32, "state total i":i32, "state main i":i32}
  T5 = cluster{"Time_total":dbl, "Time_run":dbl, "Time_wait":dbl}
  T6 = cluster{"Points-2":cluster{"X":sgl, "Y":sgl}[]}[]
  T7 = typedef "IMAQ Image.ctl" = refnum<image>
  T8 = cluster{"Array out":cluster{"x":dbl, "y":dbl}[]}[]
  T9 = cluster{"output high":dbl, "output low":dbl, "output":dbl}
  T10 = cluster{"stop pt array out":cluster{"X":dbl, "Y":dbl}[]}[]
  T11 = cluster{"heading_curr ":cluster{"x":dbl, "y":dbl}[]}[]
  T12 = enum16{"none", "arrow", "blue", "blue_small", "blue_dot", "blue_pushpin", "brown_small", "gray_small", "green", "green_small", "green_dot", "green_pushpin", "green_big_go", "yellow", "yellow_small", "yellow_dot", "yellow_big_pause", "yellow_pushpin", "lightblue", "lightblue_dot", "lightblue_pushpin", "orange", "orange_small", "orange_dot", "pink", "pink_dot", "pink_pushpin", "purple", "purple_small", "purple_dot", "purple_pushpin", "red", "red_small", "red_dot", "red_pushpin", "red_big_stop", "black_small", "white_small"}
  T13 = enum32{"AGV", "LIDAR", "PID", "GNSS", "Vision", "File", "Waypoint", "Joystick", "Etc"}
  T14 = cluster{"Linear Velocity (m/s)":dbl, "Angular Velocity (rad/s)":dbl, "Battery Voltage":dbl}
  T15 = cluster{"state":string, "Mode":u8, "Battery V":dbl, "error High":u8, "error Low":u8}
  T16 = cluster{"Port":refnum<visa-resource-name>, "speed limits":cluster{"speed-limit":dbl, "steer-limit":dbl}, "limits":cluster{"speed limits":cluster{"max":dbl, "min":dbl}, "steer limits":cluster{"max":dbl, "min":dbl}}}
  T17 = cluster{"lookahead points":dbl, "lookahead distance":dbl}
  T18 = cluster{" turn steer speed":dbl, "move speed":dbl, "slow down factor":dbl, "adjust angle margin":dbl}
  T19 = cluster{"TIM571 IP":string, "h range":cluster{i16, i16}}
  T20 = cluster{"port":refnum<visa-resource-name>, "dt":u32, "cicle":u8, "speed":u16, "rate":u32}
  T21 = cluster{"h range":cluster{i16, i16}, "v range":cluster{i8, i8}}
  T22 = cluster{"PID gains":cluster{"proportional gain (Kc)":dbl, "integral time (Ti, min)":dbl, "derivative time (Td, min)":dbl}, "PID limits":cluster{"output high":dbl, "output low":dbl}, "dt_pid":u32}
  T23 = cluster{"Port":refnum<visa-resource-name>, "PwrPak7_heading select":string, "PwrPak7_mode select":string[]}
  T24 = typedef "IMAQdx.ctl" = refnum<k21>
  T25 = cluster{"Clamp Settings":cluster{"Contrast":i32, "Filter width":i32, "Steepness":i32, "Subsampling Ratio":u32, "Show Search Area":bool, "Show Search Lines":bool, "Show Edges Found":bool, "Show Result":bool}, "Threshold Range":cluster{"Lower value":sgl, "Upper value":sgl}, "N of Erosion 1":i32, "N of Erosion 2":i32}
  T26 = cluster{"Waypoint array":cluster{"sel":bool, "inv":bool, "path":path}[]}
  T27 = cluster{"ref waypt 0703 A \ngoal point start":cluster{"X":dbl, "Y":dbl}[]}[]
  T28 = typedef "joystick cfg.ctl" = cluster{"Type":enum16{"Logitech F710", "Xbox"}, "steer limit":cluster{"min":dbl, "max":dbl, "scale":dbl, "offset":dbl}, "speed limit":cluster{"min":dbl, "max":dbl, "pwm max":dbl}, "ID":i32, "joystick max":dbl}
  T29 = typedef "system_hw.ctl" = cluster{"AGV":enum16{"none", "ERP42", "ERP42mini", "Scout", "Ycar"}, "Lidar 1":enum16{"none", "VLP16", "TIM571", "RPLidar A2", "RPLidar A3"}, "Lidar 2":enum16{"none", "VLP16", "TIM571", "RPLidar A2", "RPLidar A3"}, "GPS":enum16{"none", "F9P", "M8P", "PwrPak7", "19X HVS"}, "Camera":enum16{"none", "C920", "C922", "GT1290C", "MS LifeCam"}, "Joystick":enum16{"none", "joystick"}}
  T30 = typedef "marker_info.ctl" = cluster{"arrLatLngActv":dbl[], "type":i32}
  T31 = typedef "gmap_fgv-cmd.ctl" = enum16{"marker type change", "save_image", "coll of points", "zoom n center markers", "add overlay reference", "read", "zoom", "set position by keyword", "set map provider", "map provider update", "create", "add marker", "clear marker", "close"}
  T32 = enum16{"Config Save", "Config Load", "LastRUN Save", "LastRUN Load"}
  T33 = cluster{"Name":string, "Color":u32, "Style":u8, "Point Style":u8, "Name Visible":bool, "Allow Drag":bool, "Annotation Mode":u32, "Plot":i32, "Index":i32, "Position":cluster{"X":dbl, "Y":dbl}, "X Scale":u32, "Y Scale":u32, "Show Arrow":bool, "Lock Name":bool, "Plot Area":i32, "Label Offset":cluster{"X":dbl, "Y":dbl}}
  T34 = enum8{"Enabled", "Disabled", "Disabled and Grayed Out"}
  T35 = typedef "error_modules.ctl" = enum16{"init", "read", "TIM571 error in", "VLP16 error in", "PwrPak7 error in"}
  T36 = typedef "log_buffq.ctl" = enum16{"create", "write", "read", "close"}
  T37 = typedef "agv_cmd_v.ctl" = enum16{"write limit", "init stop", "write", "read"}
  T38 = typedef "cmd_common.ctl" = enum16{"read", "write"}
  T39 = cluster{"VLP16 cfg":refnum<vi>, "TIM571 cfg":refnum<vi>, "PID cfg":refnum<vi>, "AGV cfg":refnum<vi>, "GPS cfg":refnum<vi>, "camera cfg":refnum<vi>, "ybbaek copyright":refnum<vi>, "Obstacle limit cfg":refnum<vi>, "State machine cfg":refnum<vi>, "Lookahead cfg":refnum<vi>, "waypoint files cfg":refnum<vi>, "Vison cfg":refnum<vi>, "RPLidar cfg":refnum<vi>, "point all":refnum<vi>, "HW info":refnum<vi>, "Joystick cfg":refnum<vi>}
  T40 = cluster{"VLP16 cfg":cluster{"h range":cluster{i16, i16}, "v range":cluster{i8, i8}}, "TIM571 cfg":cluster{"IP":string, "h range":cluster{i16, i16}}, "AGV cfg":cluster{"Port":refnum<visa-resource-name>, "speed limits":cluster{"limit_linear-v":dbl, "limit_angular-v":dbl}, "limits":cluster{"speed limits":cluster{"max":dbl, "min":dbl}, "steer limits":cluster{"max":dbl, "min":dbl}}}, "GPS cfg":cluster{"PwrPak7 Port":refnum<visa-resource-name>, "heading select":string, "mode select":string[]}, "PID cfg":cluster{"PID gains":cluster{"proportional gain (Kc)":dbl, "integral time (Ti, min)":dbl, "derivative time (Td, min)":dbl}, "PID limits":cluster{"output high":dbl, "output low":dbl}, "dt pid":u32}, "Lookahead cfg":cluster{"lookahead pts n":dbl, "lookahead distance":dbl}, "Obstacle limit range":cluster{"RL range":dbl, "Point limit":u16}, "State machine parameter":cluster{"angle adjust limit":dbl}, "waypoint group":cluster{"Waypoint array":cluster{"sel":bool, "inv":bool, "path":path}[]}, "State machine cfg":cluster{" turn angular speed":dbl, "move linear speed":dbl, "decrease factor linear speed":dbl, "adjust angle margin":dbl}, "camera cfg":cluster{"Port":T24, "Camera file":path}, "ROI-clamp":cluster{"Global Rectangle":i32[], "Contours":cluster{"Contour Type":u32, "ROI Type":u32, "Points":i32[]}[]}, "x-center":dbl, "Image Size":cluster{"x":i32, "y":i32}, "Angle deg":sgl, "Vison cfg":cluster{"Clamp Settings":cluster{"Contrast":i32, "Filter width":i32, "Steepness":i32, "Subsampling Ratio":u32, "Show Search Area":bool, "Show Search Lines":bool, "Show Edges Found":bool, "Show Result":bool}, "Range":cluster{"Lower value":sgl, "Upper value":sgl}, "N of Erosion 1":i32, "N of Erosion 2":i32}, "RPLidar cfg":cluster{"port":refnum<visa-resource-name>, "dt":u32, "update":u8, "speed":u16, "rate ":u32}, "HW info":T29, "Joystick cfg":T28}
  T41 = cluster{"Name":string, "Color":u32, "Style":u8, "Point Style":u8, "Name Visible":bool, "Allow Drag":bool, "Annotation Mode":u32, "Plot":i32, "Index":i32, "Position":cluster{"X":dbl, "Y":dbl}, "X Scale":u32, "Y Scale":u32, "Show Arrow":bool, "Lock Name":bool, "Plot Area":i32, "Label Offset":cluster{"X":dbl, "Y":dbl}}[]
  T42 = cluster{"AGV":T2, "AGV Estop":T2, "Obstacle":T2, "Heading":T2, "Waypt":T2, "GNSS":T2, "VLP16":T2, "Cam":T2, "RPLidar":T2, "Joystick":T2}
  T43 = cluster{"Global Rectangle":i32[], "Contours":cluster{"Contour Type":u32, "ROI Type":u32, "Points":i32[]}[]}
  T44 = cluster{"Lat":refnum<vi>, "Lon":refnum<vi>, "Lat_DbClk":refnum<vi>, "Lon_DbClk":refnum<vi>, "zoom":refnum<vi>, "PinDropMrkr":refnum<vi>}
  T45 = typedef "gmap_info.ctl" = cluster{"Zoon_info":cluster{"MaxZoom":dbl, "MinZoom":dbl, "Zoom":dbl}, "arrOverlayNames":string[], "MapProvider":string}
  T46 = typedef "gps-databuf.ctl" = enum16{"read", "write"}
  T47 = typedef "obstacle_info.ctl" = enum16{"init", "read", "obstacle status in", "write limit", "inrange pt-n"}
  T48 = typedef "pid-in-params.ctl" = enum16{"read", "write"}
  T49 = typedef "waypoint_buf.ctl" = enum16{"clear", "write", "read"}
  T50 = typedef "pid-status.ctl" = enum16{"read", "wirte pid dt", "wirte pid output"}
  T51 = typedef "pid-cfg.ctl" = enum16{"read", "write pid gain", "write pid limit", "pid dt"}
  T52 = cluster{"rawdata":string, "GPS Data":cluster{"Latitude":cluster{"Valid?":bool, "Latitude (Deg)":dbl}, "Longitude":cluster{"Valid?":bool, "Longitude (Deg)":dbl}, "Height":cluster{"Valid?":bool, "Height (m)":dbl}, "Undulation":cluster{"Valid?":bool, "Undulation(m)":dbl}, "North Vel":cluster{"Valid?":bool, "North Vel (m/s)":dbl}, "East Vel":cluster{"Valid?":bool, "East Vel (m/s)":dbl}, "Up Vel":cluster{"Valid?":bool, "Up Vel (m/s)":dbl}, "Roll":cluster{"Valid?":bool, "Roll (degrees)":dbl}, "Pitch":cluster{"Valid?":bool, "Pitch (degrees)":dbl}, "Azimuth":cluster{"Valid?":bool, "Azimuth (degrees)":dbl}, "Lat deviation":cluster{"Valid?":bool, "Lat deviation (m)":dbl}, "Long deviation":cluster{"Valid?":bool, "Long deviation (m)":dbl}, "Height deviation":cluster{"Valid?":bool, "Height deviation (m)":dbl}, "North vel deviation":cluster{"Valid?":bool, "North vel deviation (m/s)":dbl}, "East vel deviation":cluster{"Valid?":bool, "East vel deviation (m/s)":dbl}, "Up vel deviation":cluster{"Valid?":bool, "Up vel deviation (m/s)":dbl}, "Roll deviation":cluster{"Valid?":bool, "Roll deviation (degrees)":dbl}, "Pitch deviation":cluster{"Valid?":bool, "Pitch deviation (degrees)":dbl}, "Azimuth deviation":cluster{"Valid?":bool, "Azimuth deviation (degrees)":dbl}, "Ext sol status":cluster{"Valid?":bool, "Ext sol status":dbl}}, "Heading":dbl, "utm-1":cluster{"XN":dbl, "YE":dbl}}
  T53 = cluster{"total time":dbl, "run time":dbl, "wait time":dbl}
  T54 = cluster{"deg_agv-lookahead":dbl, "deg_waypoint":dbl, "deg_gap":dbl, "deg_target":dbl, "pid output":dbl, "distance-gap_out":dbl}
  T55 = cluster{"lookahead pt n":dbl, "lookahead distance":dbl}
  T56 = cluster{"System Feedback":cluster{"system state":string, "Control Mode":u8, "Battery Voltage":dbl, "error code High":u8, "error code Low":u8}, "Motion Feedback":cluster{"Linear Velocity (m/s)":dbl, "Angular Velocity (rad/s)":dbl}}
  T57 = cluster{"system state":string, "Control Mode":u8, "Battery Voltage":dbl, "error code High":u8, "error code Low":u8}
  T58 = cluster{"Linear Velocity (m/s)":dbl, "Angular Velocity (rad/s)":dbl}
  T59 = cluster{"start point":cluster{"x":dbl, "y":dbl}, "stop point":cluster{"x":dbl, "y":dbl}}
  T60 = cluster{"progress_curr":dbl, "progress_all":dbl, "distance_left":dbl, "distance_all":dbl}
  T61 = cluster{"output high":dbl, "output low":dbl, "pid output":dbl}
  T62 = cluster{"total time":dbl, "run time":dbl, "pause time":dbl}
  T63 = typedef "mapinfo.ctl" = cluster{"GmapDotNet":refnum<k24>, "mapprovider_info":cluster{"index":i32, "dotnetrefs":refnum<k24>, "Name":string}[]}
  T64 = cluster{"index":i32, "dotnetrefs":refnum<k24>, "Name":string}[]
  T65 = cluster{"index":i32, "dotnetrefs":refnum<k24>, "Name":string}
  T66 = typedef "data.ctl" = cluster{"Drive_value":cluster{"F/B":enum16{"Go", "N", "Back"}, "Speed":u16, "Steer":i16, "A/M":enum16{"Brake", "Auto", "Manual"}, "Brake":u8}}
  T67 = enum16{"none", "ERP42", "ERP42mini", "Scout", "Ycar"}
  T68 = enum16{"none", "VLP16", "TIM571", "RPLidar A2", "RPLidar A3"}
  T69 = enum16{"none", "F9P", "M8P", "PwrPak7", "19X HVS"}
  T70 = enum16{"none", "C920", "C922", "GT1290C", "MS LifeCam"}
  T71 = cluster{"latlong out":dbl[], "PinDropMrkr":enum16{"none", "arrow", "blue", "blue_small", "blue_dot", "blue_pushpin", "brown_small", "gray_small", "green", "green_small", "green_dot", "green_pushpin", "green_big_go", "yellow", "yellow_small", "yellow_dot", "yellow_big_pause", "yellow_pushpin", "lightblue", "lightblue_dot", "lightblue_pushpin", "orange", "orange_small", "orange_dot", "pink", "pink_dot", "pink_pushpin", "purple", "purple_small", "purple_dot", "purple_pushpin", "red", "red_small", "red_dot", "red_pushpin", "red_big_stop", "black_small", "white_small"}}
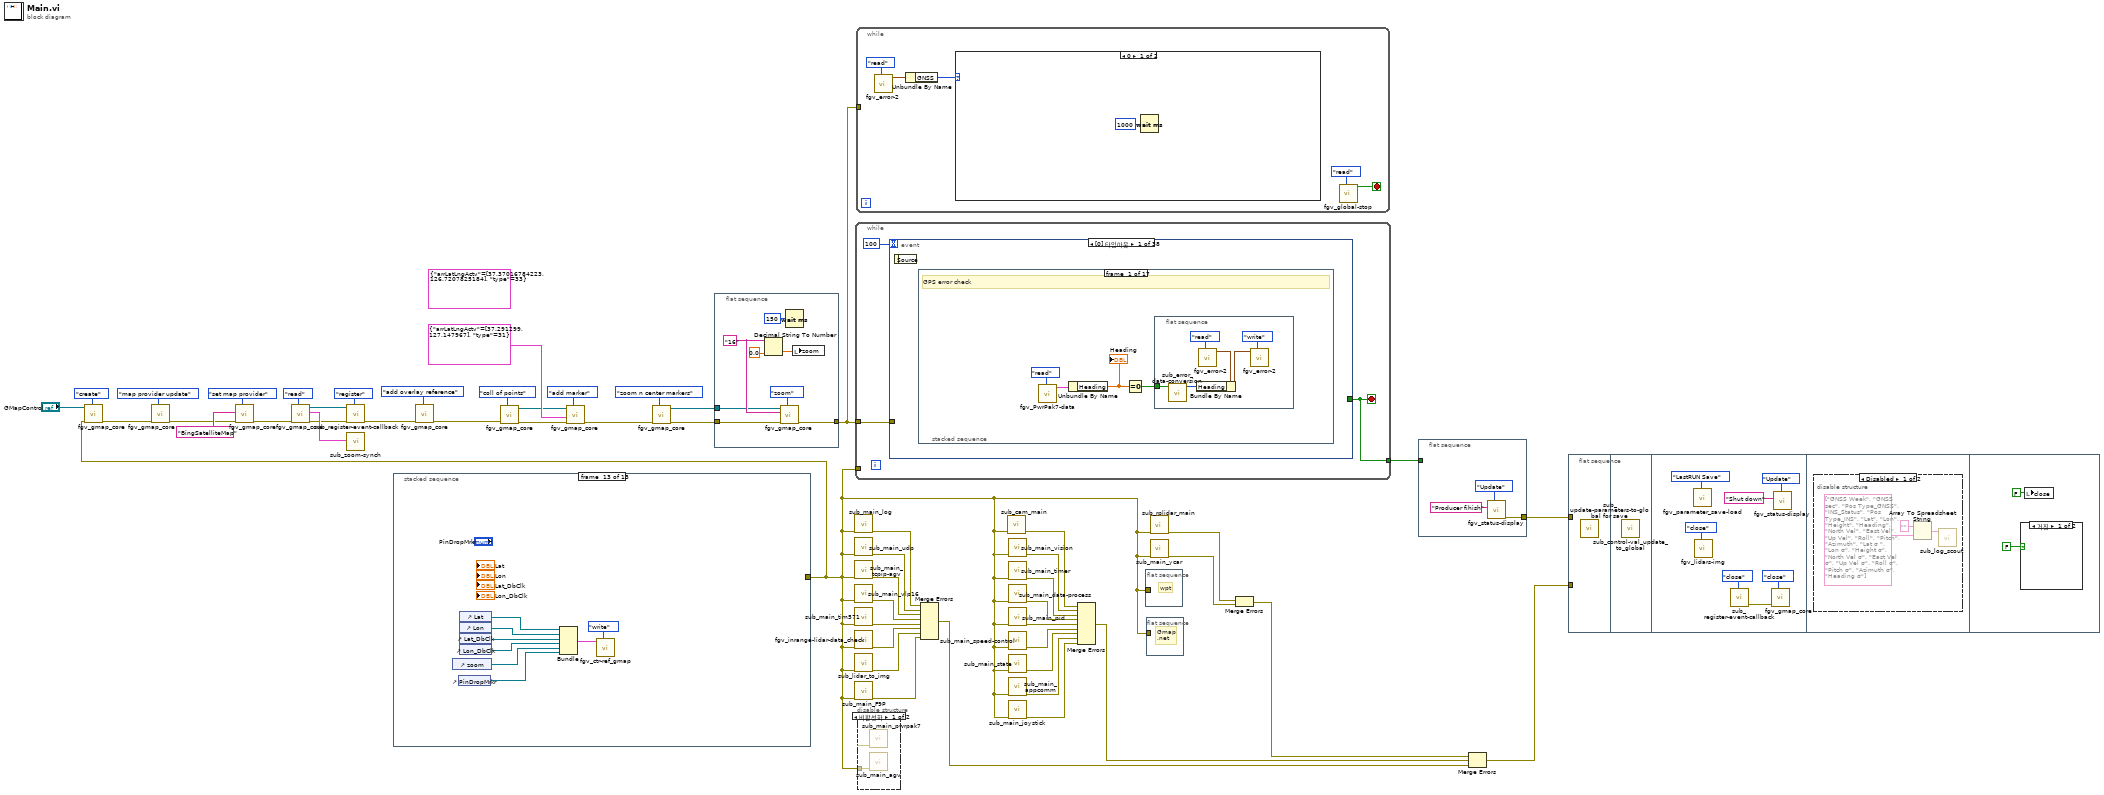
[diagram p0: block diagram]
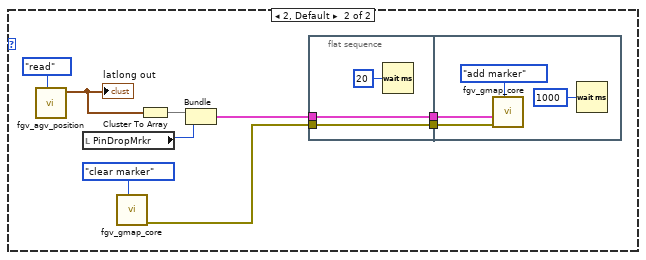
[diagram p2: hidden frame]
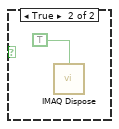
[diagram p5: hidden frame]
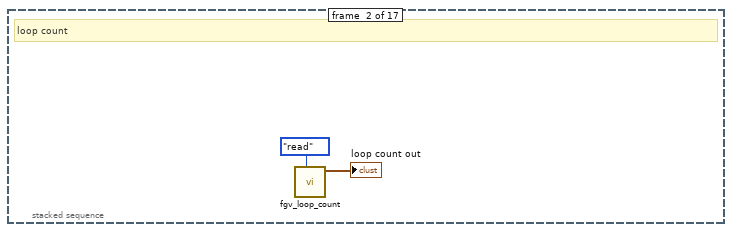
[diagram p6: hidden frame]
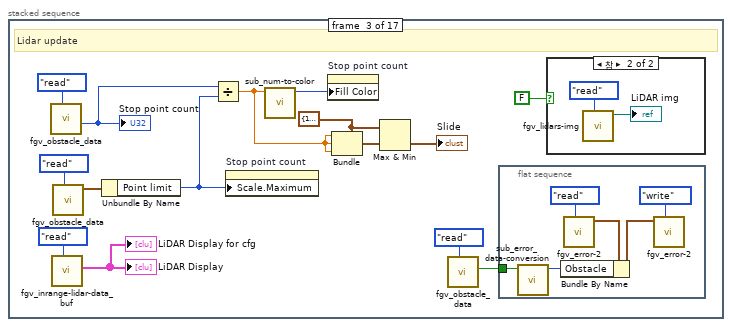
[diagram p7: hidden frame]
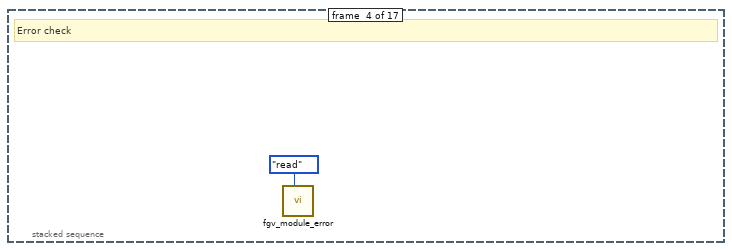
[diagram p9: hidden frame]
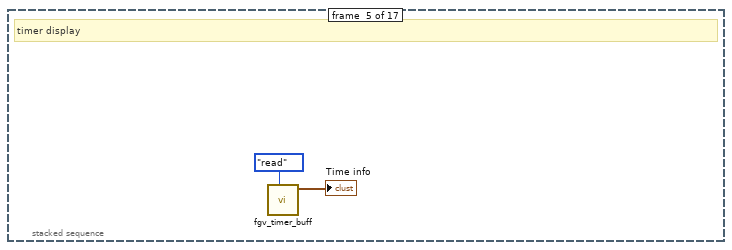
[diagram p10: hidden frame]
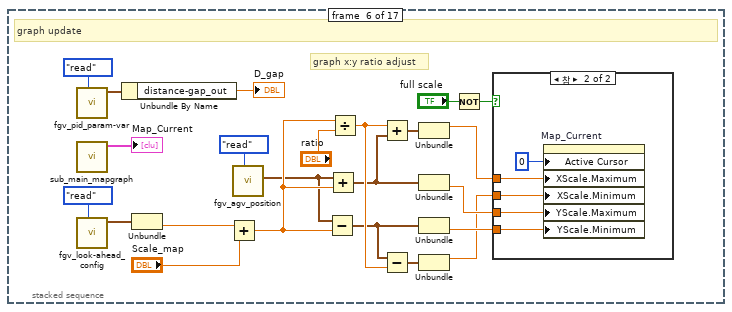
[diagram p11: hidden frame]
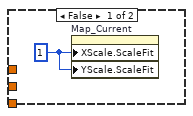
[diagram p12: hidden frame]
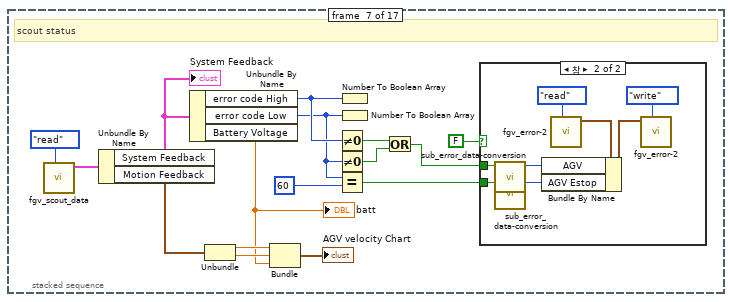
[diagram p13: hidden frame]
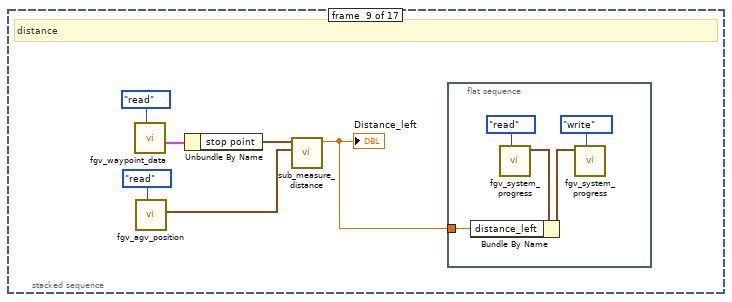
[diagram p16: hidden frame]
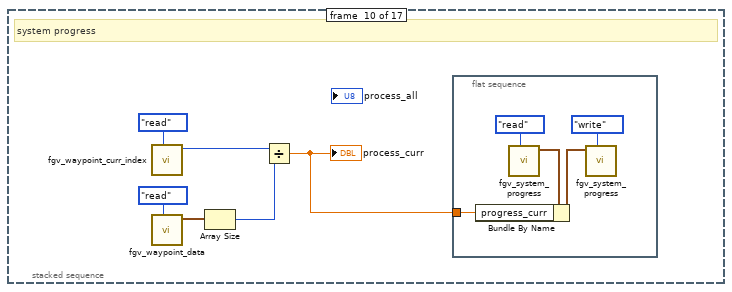
[diagram p17: hidden frame]
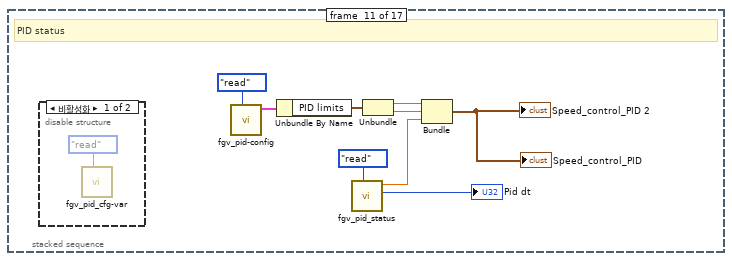
[diagram p18: hidden frame]
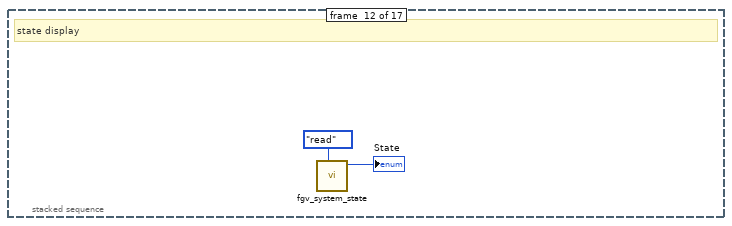
[diagram p20: hidden frame]
diagram:
  (unwired) T30 {"arrLatLngActv"=[37.37016784223, 126.7207825184], "type"=33} ("marker_info")
  n1 = stacked-sequence {
    tunnel: [_ _ _ _ w97 _ _ _ _ _ _ _ _] -> w1
    frame #0 {
      # "conrol ref - Parameter loading from file"
      n2 = control-ref of="GMapControl"() -> ()  [unwired: 1 out]
      n3 = control-ref of="point all"() -> (w58:refnum<vi>)
      n4 = control-ref of="VLP16 cfg"() -> (w63:refnum<vi>)
      n5 = control-ref of="TIM571 cfg"() -> (w71:refnum<vi>)
      n6 = control-ref of="PID cfg"() -> (w70:refnum<vi>)
      n7 = control-ref of="AGV cfg"() -> (w69:refnum<vi>)
      n8 = control-ref of="GPS cfg"() -> (w68:refnum<vi>)
      n9 = control-ref of="camera cfg"() -> (w62:refnum<vi>)
      n10 = control-ref of="Obstacle limit cfg"() -> (w67:refnum<vi>)
      n11 = control-ref of="State machine cfg"() -> (w66:refnum<vi>)
      n12 = control-ref of="Lookahead cfg"() -> (w64:refnum<vi>)
      n13 = control-ref of="waypoint files cfg"() -> (w65:refnum<vi>)
      n14 = control-ref of="Vison cfg"() -> (w61:refnum<vi>)
      n15 = control-ref of="RPLidar cfg"() -> (w59:refnum<vi>)
      n16 = control-ref of="HW info"() -> (w57:refnum<vi>)
      n17 = control-ref of="Joystick cfg"() -> (w55:refnum<vi>)
      n18 = control-ref of="ybbaek copyright"() -> (w60:refnum<vi>)
      n19 = Bundle("VLP16 cfg"=w63, "TIM571 cfg"=w71, "PID cfg"=w70, "AGV cfg"=w69, "GPS cfg"=w68, "camera cfg"=w62, "ybbaek copyright"=w60, "Obstacle limit cfg"=w67, "State machine cfg"=w66, "Lookahead cfg"=w64, "waypoint files cfg"=w65, "Vison cfg"=w61, "RPLidar cfg"=w59, "point all"=w58, "HW info"=w57, "Joystick cfg"=w55) -> (w53:T39)  [unwired: 1 in]
      n20 = call "fgv_ctrl-ref.vi"("cmd"=enum16{"write", "read"}."write", "ref"=w53) -> ("error out"=w54:errorcluster)  [unwired: 8 in, 1 out]
      n21 = flat-sequence {
        tunnel: w54 -> [_]
        frame #0 {
          n22 = call "fgv_parameter_save-load.vi"("ctl"=T32."LastRUN Load") -> ()  [unwired: 9 in, 2 out]
        }
        frame #1 {
          n23 = call "sub_control-val_update_from_global.vi"() -> ()  [unwired: 12 in]
        }
      }
    }
    frame #1 {
      # "log init"
      n24 = flat-sequence {
        frame #0 {
          n25 = call "sub_log_fine-name.vi"() -> ()  [unwired: 12 in]
        }
        frame #1 {
          n26 = disable-structure shown="비활성화" {
            frame Disabled {
              n27 = global read "global_setting.vi" "Settings"() -> (w74:T40)
              n28 = Flatten To XML(anything=w74) -> (xml string=w73:string)
              n29 = call "sub_log_basic.vi"("desc"=w73, "Title"="log_settings") -> ()  [unwired: 9 in, 1 out]
            }
            frame Enabled {
            }
          }
        }
        frame #2 {
          n30 = call "sub_check-ip.vi"() -> ("ip output"=w76:string, "standard output"=w81:string)  [unwired: 10 in]
          n31 = call "sub_log_basic.vi"("desc"=w81, "Title"="ipstatus") -> ()  [unwired: 9 in, 1 out]
          n32 = call "fgv_system_info.vi"("cmd"=enum16{"read", "write"}."read") -> ("info_out"=w78:cluster{"ip":string})  [unwired: 10 in]
          n33 = Bundle By Name(cluster=w78, "ip"=w76) -> (w77:cluster{"ip":string})
          n34 = call "fgv_system_info.vi"("cmd"=enum16{"read", "write"}."read", "info"=w77) -> ()  [unwired: 9 in, 1 out]
        }
      }
    }
    frame #2 {
      w83 = FALSE ("close")
      w85 = T34."Disabled and Grayed Out" ("비활성화")
      # "etc"
      n35 = case shown="참" FALSE {
        frame False {
        }
        frame True {
          w86 = TRUE ("Name Visible")
          n36 = Bundle By Name(cluster=T33 {"Name"="", "Color"=0, "Style"=0, "Point Style"=0, "Name Visible"=FALSE, "Allow Drag"=FALSE, "Annotation Mode"=0, "Plot"=0, "Index"=0, "Position"={"X"=0.0, "Y"=0.0}, "X Scale"=0, "Y Scale"=0, "Show Arrow"=TRUE, "Lock Name"=FALSE, "Plot Area"=0, "Label Offset"={"X"=0.0, "Y"=0.0}} ("원소"), "Color"=u32 0, "Name Visible"=w86, "Lock Name"=w86) -> (w89:T33)
          n37 = Build Array(w89) -> (w90:T41)
          n38 = property on="Map_Total" class="XYGraph (엄격한)"("AnntList"=w90) -> ()  [unwired: 2 in, 2 out]
        }
      }
      n39 = local write "close"(w83) -> ()
      n40 = local write "start-stop"(w83) -> ()
      n41 = property on="start-stop" class="Bool (엄격한)"("DisabledEnum"=w85) -> ()  [unwired: 2 in, 2 out]
      n42 = property on="pause-resume" class="Bool (엄격한)"("DisabledEnum"=w85) -> ()  [unwired: 2 in, 2 out]
    }
    frame #3 {
      # "display monitor"
      n43 = flat-sequence {
        frame #0 {
          n44 = control-ref of="System status"() -> (w95:refnum<vi>)
          n45 = call "fgv_status-display.vi"("Mode"=enum16{"Initial", "Update", "Clear"}."Initial", "System Log"=w95) -> ("error out"=w94:errorcluster)  [unwired: 9 in]
          n46 = call "fgv_status-display.vi"("Mode"=enum16{"Initial", "Update", "Clear"}."Update", "error in"=w94, "title"="System start" ("String in 1")) -> ()  [unwired: 8 in, 1 out]
        }
      }
    }
    frame #4 {
      # "Log in account"
      n47 = case shown="거짓" FALSE {
        tunnel: [T34."Enabled" ("비활성화") w100] -> w96
        frame False {
        }
        frame True {
          n48 = call "login simple.vi"() -> ("pass - fail"=w101:bool)  [unwired: 11 in]
          n49 = case shown="거짓" w101 {
            tunnel: [T34."Disabled and Grayed Out" ("비활성화") T34."Enabled" ("비활성화")] -> w100
            frame False {
            }
            frame True {
            }
          }
        }
      }
      n50 = property on="Checking" class="Bool"("DisabledEnum"=w96) -> (error out=w97:errorcluster)  [unwired: 2 in, 1 out]
    }
    frame #5 {
      # "total map update"
      n51 = call "fgv_waypoint_total.vi"("cmd"=enum16{"write", "read"}."read") -> ("waypoint total out"=w106:cluster{"waypt":cluster{"X":dbl, "Y":dbl}[]}[])  [unwired: 10 in]
      n52 = for {
        shift-right: [w108] -> w107
        shift-left: T27 [] -> [w109]
        tunnel: w106 -> [w110] mode=indexing
        n53 = Build Array (concatenate)(w109, w110) -> (w108:cluster{"waypt":cluster{"X":dbl, "Y":dbl}[]}[])
      }
      n54 = local write "Map_Total"(w107) -> ()
    }
    frame #6 {
      # "hw prod cons q creation"
      n55 = disable-structure shown="비활성화" {
        frame Disabled {
          n56 = call "fgv_q_agv.vi"("cmd"=enum16{"create", "write", "read", "close"}."create") -> ()  [unwired: 9 in, 2 out]
          n57 = call "fgv_erp42_q.vi"("cmd"=enum16{"create", "write", "read", "close"}."create") -> ()  [unwired: 9 in, 2 out]
          n58 = call "fgv_erp42mini-232_q.vi"("cmd"=enum16{"create", "write", "read", "close"}."create") -> ()  [unwired: 9 in, 2 out]
          n59 = call "fgv_q_PwrPak7.vi"("cmd"=enum16{"create", "write", "read", "close"}."create") -> ()  [unwired: 9 in, 2 out]
        }
        frame Enabled {
        }
      }
      n60 = call "fgv_pc_cam_q.vi"("cmd"=enum16{"create", "write", "read", "close"}."create") -> ()  [unwired: 9 in, 2 out]
      n61 = call "fgv_q_vlp16.vi"("cmd"=enum16{"create", "write", "read", "close"}."create") -> ()  [unwired: 9 in, 2 out]
      n62 = call "fgv_rplidar_232_q.vi"("cmd"=enum16{"create", "write", "read", "close"}."create") -> ()  [unwired: 9 in, 2 out]
      n63 = call "fgv_F9P_q.vi"("cmd"=enum16{"create", "write", "read", "close"}."create") -> ()  [unwired: 9 in, 2 out]
      n64 = call "fgv_q_tim571.vi"("cmd"=enum16{"create", "write", "read", "close"}."create") -> ()  [unwired: 9 in, 2 out]
      n65 = call "fgv_ycar_q.vi"("cmd"=enum16{"create", "write", "read", "close"}."create") -> ()  [unwired: 9 in, 2 out]
      n66 = call "fgv_q_joystick.vi"("cmd"=enum16{"create", "write", "read", "close"}."create") -> ()  [unwired: 9 in, 2 out]
    }
    frame #7 {
      # "not using"
      # "fgv q"
      n67 = disable-structure shown="비활성화" {
        frame Disabled {
          n68 = call "fgv_erp42_data.vi"("cmd"=enum16{"init", "read", "write"}."init") -> ()  [unwired: 8 in, 3 out]
        }
        frame Enabled {
        }
      }
      n69 = call "fgv_stop-point_databuf.vi"("cmd"=enum16{"clear", "write", "read"}."clear") -> ()  [unwired: 10 in, 1 out]
      n70 = call "fgv_local-stop_agv.vi"("cmd"=enum16{"ini", "read", "stop"}."ini") -> ()  [unwired: 10 in, 1 out]
      n71 = call "fgv_global-stop.vi"("cmd"=enum16{"init", "stop", "read"}."init") -> ()  [unwired: 10 in, 1 out]
      n72 = call "fgv_module_error.vi"("cmd"=error_modules."init") -> ()  [unwired: 8 in, 3 out]
      n73 = call "fgv_error-2.vi"("cmd"=enum16{"init", "read", "write"}."init") -> ()  [unwired: 9 in, 2 out]
      n74 = call "fgv_logbuff_q.vi"("cmd"=log_buffq."create") -> ()  [unwired: 9 in, 2 out]
      n75 = call "fgv_lane_slope-info.vi"("cmd"=enum16{"ini", "read", "write"}."ini") -> ()  [unwired: 8 in, 3 out]
      n76 = call "fgv_joystick-info.vi"("init"=enum16{"enable", "init", "read", "write"}."init") -> ()  [unwired: 7 in, 4 out]
      n77 = call "fgv_loop_count.vi"("cmd"=enum16{"init", "read", "write"}."init") -> ()  [unwired: 9 in, 2 out]
      n78 = call "fgv_system_state.vi"("cmd"=enum16{"init", "read", "write"}."init") -> ()  [unwired: 9 in, 2 out]
      n79 = call "fgv_lidars-img.vi"("cmd"=enum16{"create", "read", "close"}."create") -> ()  [unwired: 10 in, 1 out]
      n80 = call "sub_system_pause-condition.vi"("cmd"=enum16{"pause", "go", "read"}."pause") -> ()  [unwired: 10 in, 1 out]
      n81 = call "sub_hw-err-checking.vi"("cmd"=enum16{"write", "read", "init"}."init") -> ()  [unwired: 10 in, 1 out]
      n82 = call "fgv_lidars-databuf.vi"("cmd"=enum16{"ini img arr", "write", "read"}."ini img arr") -> ()  [unwired: 9 in, 2 out]
      n83 = call "fgv_hw-err.vi"("cmd"=enum16{"ini", "read", "write"}."ini") -> ()  [unwired: 10 in, 1 out]
    }
    frame #8 {
      # "agv"
      n84 = call "fgv_agv_cmd-val.vi"("cmd"=agv_cmd_v."init stop") -> ()  [unwired: 9 in, 2 out]
      n85 = call "fgv_agv_speedsteer-common.vi"("cmd"=enum16{"init", "read", "write"}."init") -> ()  [unwired: 9 in, 2 out]
      n86 = disable-structure shown="비활성화" {
        frame Disabled {
          n87 = call "fgv_erp42_opval.vi"("cmd"=enum16{"read", "write", "ini"}."ini") -> ()  [unwired: 10 in, 1 out]
          n88 = call "fgv_erp42mini-opval.vi"("cmd"=enum16{"ini", "read", "wirte"}."ini") -> ()  [unwired: 10 in, 1 out]
          n89 = call "fgv_hw-info.vi"("cmd"=enum16{"write", "read"}."write") -> ()  [unwired: 10 in, 1 out]
        }
        frame Enabled {
        }
      }
    }
    frame #9 {
      # "way point"
      n90 = call "fgv_waypoint_config.vi"("cmd"=enum16{"read", "write"}."read") -> ("waypoint files cfg out"=w154:T26)  [unwired: 10 in]
      n91 = call "sub_waypoints_upload.vi"("waypoint group"=w154) -> ("waypt error"=w143:bool, "waypoint all"=w155:cluster{"XY 그래프":cluster{"X":dbl, "Y":dbl}[]}[])  [unwired: 9 in]
      n92 = call "fgv_waypoint_total.vi"("cmd"=enum16{"write", "read"}."write", "waypoint total in"=w155) -> ("waypoint total out"=w150:cluster{"waypt":cluster{"X":dbl, "Y":dbl}[]}[])  [unwired: 9 in]
      n93 = call "sub_error_data-conversion.vi"("error status"=w143) -> ("error conversion out"=w144:T2)  [unwired: 9 in, 1 out]
      n94 = Build Array (concatenate)(cluster{"stop pt array out":cluster{dbl, dbl}[]} {"stop pt array out"=[]} ("출력 클러스터"), w150) -> (w149:cluster{"waypt":cluster{"X":dbl, "Y":dbl}[]}[])
      n95 = call "fgv_error-2.vi"("cmd"=enum16{"init", "read", "write"}."read") -> ("Error cluster out"=w147:T42)  [unwired: 9 in, 1 out]
      n96 = Bundle By Name(cluster=w147, "Waypt"=w144) -> (w148:T42)
      n97 = local write "Total map cfg"(w149) -> ()
      n98 = call "fgv_error-2.vi"("cmd"=enum16{"init", "read", "write"}."write", "Error cluster"=w148) -> ()  [unwired: 8 in, 2 out]
    }
    frame #10 {
      # "stop point"
      n99 = call "fgv_stop-point_config.vi"("cmd"=enum16{"read", "write"}."write", "config value"="stop point config") -> ()  [unwired: 9 in, 1 out]
      n100 = call "fgv_timer_stop-point.vi"("cmd"=enum16{"check", "start", "pause"}."start") -> ()  [unwired: 8 in, 3 out]
      n101 = call "fgv_stop-point_databuf.vi"("cmd"=enum16{"clear", "write", "read"}."clear") -> ()  [unwired: 10 in, 1 out]
    }
    frame #11 {
      # "vision"
      n102 = call "fgv_imgbuf_raw.vi"("cmd"=enum16{"create", "close", "write", "read"}."create") -> ()  [unwired: 9 in, 2 out]
      n103 = call "fgv_imgbuf_processing.vi"("cmd"=enum16{"create", "close", "write", "read"}."create") -> ()  [unwired: 9 in, 2 out]
      n104 = call "fgv_imgbuf_binary.vi"("cmd"=enum16{"create", "close", "write", "read"}."create") -> ()  [unwired: 9 in, 2 out]
      n105 = call "fgv_clamp_roi.vi"("cmd"=enum16{"init", "read", "write"}."read") -> ("ROI-clamp out"=w160:T43)  [unwired: 10 in]
      n106 = property on="Image_gray" class="ImageControl"("ROI"=w160) -> ()  [unwired: 2 in, 2 out]
    }
    frame #12 {
      n107 = control-ref of="zoom"() -> (w172:refnum<vi>)
      n108 = control-ref of="PinDropMrkr"() -> (w171:refnum<vi>)
      n109 = control-ref of="Lat"() -> (w168:refnum<vi>)
      n110 = control-ref of="Lon"() -> (w167:refnum<vi>)
      n111 = control-ref of="Lat_DbClk"() -> (w166:refnum<vi>)
      n112 = control-ref of="Lon_DbClk"() -> (w165:refnum<vi>)
      n113 = Bundle("Lat"=w168, "Lon"=w167, "Lat_DbClk"=w166, "Lon_DbClk"=w165, "zoom"=w172, "PinDropMrkr"=w171) -> (w170:T44)  [unwired: 1 in]
      n114 = call "fgv_ctr-ref_gmap.vi"("cmd"=cmd_common."write", "ref"=w170) -> ()  [unwired: 9 in, 1 out]
    }
  }
  n115 = call "fgv_gmap_core.vi"("cmd"=gmap_fgv-cmd."create", "error in"=w1, "GMapControl"="GMapControl") -> ("error out"=w15:errorcluster)  [unwired: 5 in, 3 out]
  n116 = call "fgv_gmap_core.vi"("cmd"=gmap_fgv-cmd."map provider update", "error in"=w15) -> ("error out"=w14:errorcluster)  [unwired: 6 in, 3 out]
  n117 = call "fgv_gmap_core.vi"(7:"cmd"=gmap_fgv-cmd."set map provider" ("cmd"), "error in"=w14, 10:"cmd"="BingSatelliteMap" ("cmd")) -> ("error out"=w13:errorcluster)  [unwired: 5 in, 3 out]
  n118 = call "fgv_gmap_core.vi"("cmd"=gmap_fgv-cmd."read", "error in"=w13) -> ("error out"=w12:errorcluster, "gmap info out"=w22:T45, "GMapControl out"=w18:refnum<k24>)  [unwired: 6 in, 1 out]
  n119 = call "sub_register-event-callback.vi"("cmd"=enum16{"register", "close"}."register", "error in"=w12, "GMapControl"=w18) -> ("error out"=w17:errorcluster)  [unwired: 8 in]
  n120 = call "sub_zoom-synch.vi"("gmap info out"=w22) -> ()  [unwired: 11 in]
  n121 = call "fgv_gmap_core.vi"("cmd"=gmap_fgv-cmd."add overlay reference", "error in"=w17) -> ("error out"=w11:errorcluster)  [unwired: 6 in, 3 out]
  n122 = call "fgv_gmap_core.vi"("cmd"=gmap_fgv-cmd."coll of points", "error in"=w11) -> ("error out"=w8:errorcluster, "GMapControl out"=w7:refnum<k24>)  [unwired: 6 in, 2 out]
  n123 = call "fgv_gmap_core.vi"("cmd"=gmap_fgv-cmd."add marker", "error in"=w8, "marker_info"=T30 {"arrLatLngActv"=[37.291299, 127.147967], "type"=31}, "GMapControl"=w7) -> ("error out"=w5:errorcluster)  [unwired: 4 in, 3 out]
  n124 = call "fgv_gmap_core.vi"("cmd"=gmap_fgv-cmd."zoom n center markers", "error in"=w5) -> ("error out"=w4:errorcluster, "GMapControl out"=w3:refnum<k24>)  [unwired: 6 in, 2 out]
  n125 = flat-sequence {
    tunnel: w4 -> [w176]
    tunnel: w3 -> [w175]
    tunnel: [w173] -> w2
    frame #0 {
      w178 = "16" ("cmd")
      n126 = Decimal String To Number(string=w178, default (0L)=0.0 ("default (0 I32)")) -> (number=w180:dbl)  [unwired: 1 in, 1 out]
      n127 = call "fgv_gmap_core.vi"(7:"cmd"=gmap_fgv-cmd."zoom" ("cmd"), "error in"=w176, 10:"cmd"=w178, "GMapControl"=w175) -> ("error out"=w173:errorcluster)  [unwired: 4 in, 3 out]
      n128 = Wait (ms)(milliseconds to wait=u32 150) -> ()  [unwired: 1 out]
      n129 = local write "zoom"(w180) -> ()
    }
  }
  n130 = call "sub_main_log.vi"("error in"=w1) -> ("error out"=w46:errorcluster)  [unwired: 10 in]
  n131 = call "sub_main_udp.vi"("error in"=w1) -> ("error out"=w50:errorcluster)  [unwired: 10 in]
  n132 = call "sub_main_tcpip-agv.vi"("error in"=w1) -> ("error out"=w49:errorcluster)  [unwired: 10 in]
  n133 = call "sub_main_vlp16.vi"("error in"=w1) -> ("error out"=w48:errorcluster)  [unwired: 10 in]
  n134 = call "sub_main_tim571.vi"("error in"=w1) -> ("error out"=w47:errorcluster)  [unwired: 10 in]
  n135 = call "fgv_inrange-lidar-data_check.vi"("error in"=w1) -> ("error out"=w40:errorcluster)  [unwired: 10 in]
  n136 = call "sub_lidar_to_img.vi"("error in"=w1) -> ("error out"=w39:errorcluster)  [unwired: 10 in]
  n137 = call "sub_main_F9P.vi"("error in"=w1) -> ("error out"=w38:errorcluster)  [unwired: 10 in]
  n138 = while {
    tunnel: w1 -> [_]
    tunnel: [w183] -> w52
    tunnel: w2 -> [w181]
    stop <- w183 stop-if-true
    n139 = event shown="[0] 타임아웃" {
      selector: _ -> [_ _ _ _ _ _ _ _ _ _ _ _ _ _ _ _ _ _ _ _ _ _ _ _ _ _ _ _ _ _ _ _ _ _ _ _ _ _]
      dyn-events: _ -> [_ _ _ _ _ _ _ _ _ _ _ _ _ _ _ _ _ _ _ _ _ _ _ _ _ _ _ _ _ _ _ _ _ _ _ _ _ _]
      timeout: 100 -> [_ _ _ _ _ _ _ _ _ _ _ _ _ _ _ _ _ _ _ _ _ _ _ _ _ _ _ _ _ _ _ _ _ _ _ _ _ _]
      tunnel: [_ _ _ _ _ _ _ _ _ _ _ _ _ _ _ _ _ _ _ _ _ _ _ _ _ _ _ _ _ _ _ _ _ _ _ w547 _ _] -> w183
      tunnel: w181 -> [_ _ _ _ _ _ _ _ _ _ _ _ _ _ _ _ _ _ _ _ _ _ _ _ _ _ _ _ _ _ _ _ _ _ _ _ _ _]
      event Timeout {
        n140 = event-data() -> ()  [unwired: 1 in, 1 out]
        n141 = stacked-sequence {
          frame #0 {
            # "GPS error check"
            n142 = call "fgv_PwrPak7-data.vi"("cmd"=gps-databuf."read") -> ("data cluster out"=w187:T52)  [unwired: 9 in, 1 out]
            n143 = Unbundle By Name(w187) -> ("Heading"=w186:dbl)
            "Heading" <- w186
            n144 = Equal To 0?(x=w186) -> (x = 0?=w184:bool)
            n145 = flat-sequence {
              tunnel: w184 -> [w189]
              frame #0 {
                n146 = call "sub_error_data-conversion.vi"("error status"=w189) -> ("error conversion out"=w188:T2)  [unwired: 9 in, 1 out]
                n147 = call "fgv_error-2.vi"("cmd"=enum16{"init", "read", "write"}."read") -> ("Error cluster out"=w192:T42)  [unwired: 9 in, 1 out]
                n148 = Bundle By Name(cluster=w192, "Heading"=w188) -> (w193:T42)
                n149 = call "fgv_error-2.vi"("cmd"=enum16{"init", "read", "write"}."write", "Error cluster"=w193) -> ()  [unwired: 8 in, 2 out]
              }
            }
          }
          frame #1 {
            # "loop count"
            n150 = call "fgv_loop_count.vi"("cmd"=enum16{"init", "read", "write"}."read") -> ("loop count out"=→"loop count out":T4)  [unwired: 9 in, 1 out]
          }
          frame #2 {
            w200 = cluster{dbl, dbl, dbl} {1.0, 0.8, 0.5} ("Slide 2")
            # "Lidar update"
            n151 = call "fgv_obstacle_data.vi"("cmd"=obstacle_info."read") -> ("inrange pt-n out"=w204:u32)  [unwired: 7 in, 3 out]
            "Stop point count" <- w204
            n152 = call "fgv_inrange-lidar-data_buf.vi"("cmd"=enum16{"read", "write"}."read") -> ("in range data new out"=→"LiDAR Display" →"LiDAR Display for cfg":T8)  [unwired: 9 in, 1 out]
            n153 = call "fgv_obstacle_data.vi"("cmd"=obstacle_info."read") -> ("limit out"=w205:cluster{"RL range":dbl, "Point limit":u16})  [unwired: 7 in, 3 out]
            n154 = Unbundle By Name(w205) -> ("Point limit"=w203:u16)
            n155 = Divide(x=w204, y=w203) -> (x/y=w198:dbl)
            n156 = property on="Stop point count" class="Slide (엄격한)"("Scale.Maximum"=w203) -> ()  [unwired: 2 in, 2 out]
            n157 = call "sub_num-to-color.vi"("ratio"=w198) -> ("color num"=w202:u32)  [unwired: 10 in]
            n158 = property on="Stop point count" class="Slide (엄격한)"("Fill Color"=w202) -> ()  [unwired: 2 in, 2 out]
            n159 = Bundle(cluster=w200, w198, w198, w198) -> (w201:cluster{dbl, dbl, dbl})
            n160 = Max & Min(x=w200, y=w201) -> (min(x,y)=→"Slide":cluster{dbl, dbl, dbl})  [unwired: 1 out]
            n161 = call "fgv_obstacle_data.vi"("cmd"=obstacle_info."read") -> ("obstacle out"=w209:bool)  [unwired: 7 in, 3 out]
            n162 = flat-sequence {
              tunnel: w209 -> [w213]
              frame #0 {
                n163 = call "sub_error_data-conversion.vi"("error status"=w213) -> ("error conversion out"=w214:T2)  [unwired: 9 in, 1 out]
                n164 = call "fgv_error-2.vi"("cmd"=enum16{"init", "read", "write"}."read") -> ("Error cluster out"=w217:T42)  [unwired: 9 in, 1 out]
                n165 = Bundle By Name(cluster=w217, "Obstacle"=w214) -> (w218:T42)
                n166 = call "fgv_error-2.vi"("cmd"=enum16{"init", "read", "write"}."write", "Error cluster"=w218) -> ()  [unwired: 8 in, 2 out]
              }
            }
            n167 = case shown="참" FALSE {
              frame False {
              }
              frame True {
                n168 = call "fgv_lidars-img.vi"("cmd"=enum16{"create", "read", "close"}."read") -> ("New Image"=→"LiDAR img":T7)  [unwired: 10 in]
              }
            }
          }
          frame #3 {
            # "Error check"
            n169 = call "fgv_module_error.vi"("cmd"=error_modules."read") -> ()  [unwired: 8 in, 3 out]
          }
          frame #4 {
            # "timer display"
            n170 = call "fgv_timer_buff.vi"("cmd"=enum16{"write", "read"}."read") -> ("time_status out"=→"Time info":T53)  [unwired: 10 in]
          }
          frame #5 {
            # "graph x:y ratio adjust"
            # "graph update"
            n171 = call "fgv_pid_param-var.vi"("cmd"=pid-in-params."read") -> ("pid-var_output"=w225:T54)  [unwired: 10 in]
            n172 = call "sub_main_mapgraph.vi"() -> ("graph ui array"=→"Map_Current":T11)  [unwired: 11 in]
            n173 = call "fgv_look-ahead_config.vi"("cmd"=enum16{"read", "write"}."read") -> ("lookahed cfg out"=w240:T55)  [unwired: 10 in]
            n174 = Unbundle By Name(w225) -> ("distance-gap_out"=→"D_gap":dbl)
            n175 = Unbundle(w240) -> ("lookahead distance"=w239:dbl)  [unwired: 1 out]
            n176 = Add(x=w239, y="Scale_map") -> (x+y=w237:dbl)
            n177 = call "fgv_agv_position.vi"("cmd"=enum16{"write", "read"}."read") -> ("utm out"=w222:cluster{dbl, dbl})  [unwired: 8 in, 2 out]
            n178 = Subtract(x=w222, y=w237) -> (x-y=w233:cluster{dbl, dbl})
            n179 = Add(x=w222, y=w237) -> (x+y=w234:cluster{dbl, dbl})
            n180 = Divide(x=w237, y="ratio") -> (x/y=w235:dbl)
            n181 = Add(x=w235, y=w234) -> (x+y=w231:cluster{dbl, dbl})
            n182 = Subtract(x=w233, y=w235) -> (x-y=w232:cluster{dbl, dbl})
            n183 = Unbundle(w231) -> (w228:dbl)  [unwired: 1 out]
            n184 = Unbundle(w234) -> (w244:dbl)  [unwired: 1 out]
            n185 = Unbundle(w233) -> (w243:dbl)  [unwired: 1 out]
            n186 = Unbundle(w232) -> (w227:dbl)  [unwired: 1 out]
            n187 = Not(x="full scale") -> (.not. x?=w226:bool)
            n188 = case shown="참" w226 {
              tunnel: w244 -> [_ w250]
              tunnel: w243 -> [_ w249]
              tunnel: w228 -> [_ w247]
              tunnel: w227 -> [_ w246]
              frame False {
                w245 = u8 1 ("X Scale.Scale Fit")
                n189 = property on="Map_Current" class="XYGraph (엄격한)"("XScale.ScaleFit"=w245, "YScale.ScaleFit"=w245) -> ()  [unwired: 2 in, 2 out]
              }
              frame True {
                n190 = property on="Map_Current" class="XYGraph (엄격한)"("Active Cursor"=u32 0, "XScale.Maximum"=w247, "XScale.Minimum"=w246, "YScale.Maximum"=w250, "YScale.Minimum"=w249) -> ()  [unwired: 2 in, 2 out]
              }
            }
          }
          frame #6 {
            # "scout status"
            n191 = call "fgv_scout_data.vi"("cmd"=enum16{"write", "read"}."read") -> ("agv data out"=w263:T56)  [unwired: 10 in]
            n192 = Unbundle By Name(w263) -> ("System Feedback"=w259:T57, "Motion Feedback"=w258:T58)
            "System Feedback" <- w259
            n193 = Unbundle By Name(w259) -> ("error code High"=w261:u8, "error code Low"=w260:u8, "Battery Voltage"=w254:dbl)
            "batt" <- w254
            n194 = Unbundle(w258) -> ("Linear Velocity (m/s)"=w257:dbl, "Angular Velocity (rad/s)"=w256:dbl)
            n195 = Bundle("Linear Velocity (m/s)"=w257, "Angular Velocity (rad/s)"=w256, "Battery Voltage"=w254) -> (→"AGV velocity Chart":T14)  [unwired: 1 in]
            n196 = Not Equal To 0?(x=w261) -> (x != 0?=w264:bool)
            n197 = Not Equal To 0?(x=w260) -> (x != 0?=w265:bool)
            n198 = Equal?(x=w260, y=u8 60) -> (x = y?=w252:bool)
            n199 = Number To Boolean Array(number=w261) -> ()  [unwired: 1 out]
            n200 = Number To Boolean Array(number=w260) -> ()  [unwired: 1 out]
            n201 = Or(x=w264, y=w265) -> (x .or. y?=w253:bool)
            n202 = case shown="참" FALSE {
              tunnel: w253 -> [_ w268]
              tunnel: w252 -> [_ w267]
              frame False {
              }
              frame True {
                n203 = call "sub_error_data-conversion.vi"("error status"=w268) -> ("error conversion out"=w270:T2)  [unwired: 9 in, 1 out]
                n204 = call "sub_error_data-conversion.vi"("error status"=w267) -> ("error conversion out"=w269:T2)  [unwired: 9 in, 1 out]
                n205 = call "fgv_error-2.vi"("cmd"=enum16{"init", "read", "write"}."read") -> ("Error cluster out"=w273:T42)  [unwired: 9 in, 1 out]
                n206 = Bundle By Name(cluster=w273, "AGV"=w270, "AGV Estop"=w269) -> (w274:T42)
                n207 = call "fgv_error-2.vi"("cmd"=enum16{"init", "read", "write"}."write", "Error cluster"=w274) -> ()  [unwired: 8 in, 2 out]
              }
            }
          }
          frame #7 {
            # "ERP42 status"
          }
          frame #8 {
            # "distance"
            n208 = call "fgv_waypoint_data.vi"("cmd"=waypoint_buf."read") -> ("start-stop point"=w278:T59)  [unwired: 8 in, 2 out]
            n209 = call "fgv_agv_position.vi"("cmd"=enum16{"write", "read"}."read") -> ("utm out"=w275:cluster{dbl, dbl})  [unwired: 8 in, 2 out]
            n210 = Unbundle By Name(w278) -> ("stop point"=w277:cluster{"x":dbl, "y":dbl})
            n211 = call "sub_measure_distance.vi"("pt 2"=w275, "pt 1"=w277) -> ("distance"=w276:dbl)  [unwired: 9 in]
            "Distance_left" <- w276
            n212 = flat-sequence {
              tunnel: w276 -> [w282]
              frame #0 {
                n213 = call "fgv_system_progress.vi"("cmd"=enum16{"read", "write"}."read") -> ("progress status out"=w283:T60)  [unwired: 10 in]
                n214 = Bundle By Name(cluster=w283, "distance_left"=w282) -> (w281:T60)
                n215 = call "fgv_system_progress.vi"("cmd"=enum16{"read", "write"}."write", "progress status"=w281) -> ()  [unwired: 9 in, 1 out]
              }
            }
          }
          frame #9 {
            # "system progress"
            n216 = call "fgv_waypoint_curr_index.vi"("cmd"=enum16{"write", "read"}."read") -> ("index out"=w286:i32)  [unwired: 10 in]
            n217 = call "fgv_waypoint_data.vi"("cmd"=waypoint_buf."read") -> ("waypoint out"=w290:cluster{"x":dbl, "y":dbl}[])  [unwired: 8 in, 2 out]
            n218 = Array Size(array=w290) -> (size(s)=w287:i32)
            n219 = Divide(x=w286, y=w287) -> (x/y=w288:dbl)
            "process_curr" <- w288
            n220 = flat-sequence {
              tunnel: w288 -> [w292]
              frame #0 {
                n221 = call "fgv_system_progress.vi"("cmd"=enum16{"read", "write"}."read") -> ("progress status out"=w296:T60)  [unwired: 10 in]
                n222 = Bundle By Name(cluster=w296, "progress_curr"=w292) -> (w295:T60)
                n223 = call "fgv_system_progress.vi"("cmd"=enum16{"read", "write"}."write", "progress status"=w295) -> ()  [unwired: 9 in, 1 out]
              }
            }
          }
          frame #10 {
            # "PID status"
            n224 = disable-structure shown="비활성화" {
              frame Disabled {
                n225 = call "fgv_pid_cfg-var.vi"("cmd"=pid-cfg."read") -> ()  [unwired: 7 in, 4 out]
              }
              frame Enabled {
              }
            }
            n226 = call "fgv_pid-config.vi"("cmd"=enum16{"read", "write"}."read") -> ("PID cfg out"=w299:T22)  [unwired: 9 in, 1 out]
            n227 = Unbundle By Name(w299) -> ("PID limits"=w298:cluster{"output high":dbl, "output low":dbl})
            n228 = call "fgv_pid_status.vi"("cmd"=pid-status."read") -> ("pid dt out"=→"Pid dt":u32, "pid output"=w301:dbl)  [unwired: 8 in, 1 out]
            n229 = Unbundle(w298) -> ("output high"=w303:dbl, "output low"=w302:dbl)
            n230 = Bundle("output high"=w303, "output low"=w302, "pid output"=w301) -> (→"Speed_control_PID" →"Speed_control_PID 2":T61)  [unwired: 1 in]
          }
          frame #11 {
            # "state display"
            n231 = call "fgv_system_state.vi"("cmd"=enum16{"init", "read", "write"}."read") -> ("State out"=→"State":T1)  [unwired: 9 in, 1 out]
          }
          frame #12 {
            # "Total map update"
            n232 = call "sub_map-data_all.vi"() -> ("map-data_all"=→"Map_Total":T27)  [unwired: 11 in]
          }
          frame #13 {
            # "Error"
            n233 = call "fgv_error-2.vi"("cmd"=enum16{"init", "read", "write"}."read") -> ("Error cluster out"=→"Error Display":T42)  [unwired: 9 in, 1 out]
          }
          frame #14 {
            n234 = call "fgv_stop-point_config.vi"("cmd"=enum16{"read", "write"}."read") -> ("config value out"=w312:cluster{"stop distance":dbl, "Stop delay":dbl})  [unwired: 10 in]
            n235 = Unbundle By Name(w312) -> ("Stop delay"=w314:dbl)
            n236 = call "fgv_timer_stop-point.vi"("cmd"=enum16{"check", "start", "pause"}."check", "target time"=w314) -> ("time_status_out"=w316:T62)  [unwired: 7 in, 2 out]
            n237 = property on="stop time" class="Slide (엄격한)"("Scale.Maximum"=w314) -> ()  [unwired: 2 in, 2 out]
            n238 = Unbundle By Name(w316) -> ("total time"=→"stop time":dbl)
          }
          frame #15 {
            # "vision display"
            n239 = call "sub_lane-point_interpolation.vi"("cmd"=enum16{"init", "read", "write"}."read") -> ("graph data"=→"point all":T6)  [unwired: 7 in, 3 out]
            n240 = call "fgv_imgbuf_binary.vi"("cmd"=enum16{"create", "close", "write", "read"}."read") -> ("raw image out"=→"Image_binary" →"Image_binary 2":T7)  [unwired: 9 in, 1 out]
            n241 = call "fgv_imgbuf_raw.vi"("cmd"=enum16{"create", "close", "write", "read"}."read") -> ("Image"=→"Image_color":T7)  [unwired: 9 in, 1 out]
            n242 = call "fgv_imgbuf_processing.vi"("cmd"=enum16{"create", "close", "write", "read"}."read") -> ("Image"=→"Image_gray":T7)  [unwired: 9 in, 1 out]
          }
          frame #16 {
            n243 = call "fgv_joystick-info.vi"("init"=enum16{"enable", "init", "read", "write"}."read") -> ("v_val"=w329:cluster{dbl, dbl})  [unwired: 7 in, 3 out]
            n244 = Unbundle(w329) -> (w327:dbl, w328:dbl)
            n245 = Bundle(w328, w327) -> (w326:cluster{dbl, dbl})  [unwired: 1 in]
            n246 = Build Array(cluster{dbl, dbl} {25.0, 0.0} ("원소"), w326) -> (→"joystick":cluster{dbl, dbl}[])
          }
        }
      }
      event "SetMapProvider": Value Change {
        n247 = event-data() -> ()  [unwired: 1 in, 1 out]
        n248 = call "fgv_gmap-info.vi"("cmd"=enum16{"read", "write"}."read") -> ("mapinfo 2"=w337:T63)  [unwired: 9 in, 1 out]
        n249 = Unbundle By Name(w337) -> ("mapprovider_info"=w336:T64)
        n250 = Index Array(array=w336, index="SetMapProvider") -> (element=w334:T65)
        n251 = Unbundle By Name(w334) -> ("Name"=w333:string)
        n252 = call "fgv_gmap_core.vi"(7:"cmd"=gmap_fgv-cmd."set map provider" ("cmd"), 10:"cmd"=w333) -> ()  [unwired: 6 in, 4 out]
      }
      event "zoom-center": Value Change {
        n253 = event-data() -> ()  [unwired: 1 in, 1 out]
        n254 = call "fgv_gmap_core.vi"("cmd"=gmap_fgv-cmd."zoom n center markers") -> ()  [unwired: 7 in, 4 out]
      }
      event "zoom": Value Change {
        n255 = event-data() -> ()  [unwired: 1 in, 1 out]
        n256 = Number To Fractional String(number="zoom") -> (F-format string=w342:string)  [unwired: 3 in]
        n257 = call "fgv_gmap_core.vi"(7:"cmd"=gmap_fgv-cmd."zoom" ("cmd"), 10:"cmd"=w342) -> ()  [unwired: 6 in, 4 out]
      }
      event "Lidar graph scale": Value Change {
        n258 = event-data() -> ()  [unwired: 1 in, 1 out]
        n259 = Negate(x="Lidar graph scale") -> (-x=w344:dbl)
        n260 = property on="LiDAR Display for cfg" class="XYGraph (엄격한)"("XScale.Maximum"="Lidar graph scale", "XScale.Minimum"=w344, "YScale.Maximum"="Lidar graph scale", "YScale.Minimum"=w344) -> ()  [unwired: 2 in, 2 out]
      }
      event "camera_attrib": Value Change {
        n261 = event-data() -> ()  [unwired: 1 in, 1 out]
        n262 = call "sub_camerafile_update.vi"("camera_attrib"="camera_attrib") -> ()  [unwired: 11 in]
      }
      event "Steer": Value Change {
        n263 = event-data() -> ()  [unwired: 1 in, 1 out]
        n264 = flat-sequence {
          tunnel: "Steer" -> [w348]
          frame #0 {
            n265 = call "fgv_erp42_opval.vi"("cmd"=enum16{"read", "write", "ini"}."read") -> ("data_out"=w350:T66)  [unwired: 10 in]
            n266 = Bundle By Name(cluster=w350, "Drive_value.Steer"=w348) -> (w349:T66)
            n267 = call "fgv_erp42_opval.vi"("cmd"=enum16{"read", "write", "ini"}."write", "data_in"=w349) -> ()  [unwired: 9 in, 1 out]
          }
        }
      }
      event "Image_gray": Mouse Move {
        n268 = event-data() -> ()  [unwired: 1 in, 1 out]
        n269 = property on="Image_gray" class="ImageControl"() -> ("ROI"=w353:T43)  [unwired: 2 in, 2 out]
        n270 = call "fgv_clamp_roi.vi"("cmd"=enum16{"init", "read", "write"}."write", "ROI-clamp"=w353) -> ()  [unwired: 9 in, 1 out]
      }
      event "camera cfg": Value Change {
        n271 = event-data() -> ()  [unwired: 1 in, 1 out]
        n272 = call "fgv_cam_config.vi"("cmd"=enum16{"read", "write"}."write", "camera cfg"="camera cfg") -> ()  [unwired: 9 in, 1 out]
      }
      event "Vison cfg": Value Change {
        n273 = event-data() -> ()  [unwired: 1 in, 1 out]
        n274 = call "fgv_vision_config.vi"("cmd"=enum16{"init", "read", "write"}."write", "Vison cfg"="Vison cfg") -> ()  [unwired: 8 in, 2 out]
      }
      event "use event": Value Change {
        n275 = event-data() -> ()  [unwired: 1 in, 1 out]
        n276 = call "fgv_rplidar_232_q.vi"("cmd"=enum16{"create", "write", "read", "close"}."close") -> ()  [unwired: 9 in, 2 out]
      }
      event "stop points edit": Value Change {
        n277 = event-data() -> ()  [unwired: 1 in, 1 out]
        n278 = flat-sequence {
          frame #0 {
            n279 = call "sub_stop-point_config.vi"() -> ()  [unwired: 12 in]
          }
          frame #1 {
            n280 = call "fgv_waypoint_config.vi"("cmd"=enum16{"read", "write"}."read") -> ("waypoint files cfg out"=w368:T26)  [unwired: 10 in]
            n281 = call "sub_waypoints_upload.vi"("waypoint group"=w368) -> ("waypoint all"=w369:cluster{"XY 그래프":cluster{"X":dbl, "Y":dbl}[]}[])  [unwired: 9 in, 1 out]
            n282 = call "fgv_waypoint_total.vi"("cmd"=enum16{"write", "read"}."write", "waypoint total in"=w369) -> ("waypoint total out"=w367:cluster{"waypt":cluster{"X":dbl, "Y":dbl}[]}[])  [unwired: 9 in]
            n283 = for {
              shift-right: [w371] -> w366
              shift-left: T27 [] -> [w372]
              tunnel: w367 -> [w373] mode=indexing
              n284 = Build Array (concatenate)(w372, w373) -> (w371:cluster{"waypt":cluster{"X":dbl, "Y":dbl}[]}[])
            }
            n285 = call "fgv_stop-point_databuf.vi"("cmd"=enum16{"clear", "write", "read"}."read") -> ("all stop pts out"=w365:cluster{dbl, dbl}[])  [unwired: 10 in]
            n286 = Bundle("all stop pts out"=w365) -> (w370:cluster{"all stop pts out":cluster{dbl, dbl}[]})  [unwired: 1 in]
            n287 = Build Array (concatenate)(w370, w366) -> (w360:T27)
            n288 = local write "Total map cfg"(w360) -> ()
          }
        }
      }
      event "stop point config": Value Change {
        n289 = event-data() -> ()  [unwired: 1 in, 1 out]
        n290 = local read "stop point config"() -> (w374:cluster{"distance":dbl, "time":dbl})
        n291 = call "fgv_stop-point_config.vi"("cmd"=enum16{"read", "write"}."write", "config value"=w374) -> ()  [unwired: 9 in, 1 out]
      }
      event "test waypoint": Value Change {
        n292 = event-data() -> ()  [unwired: 1 in, 1 out]
        n293 = flat-sequence {
          frame #0 {
            n294 = disable-structure shown="비활성화" {
              frame Disabled {
                n295 = local read "waypoint files cfg"() -> (w376:T26)
                n296 = call "fgv_waypoint_config.vi"("cmd"=enum16{"read", "write"}."write", "waypoint files cfg"=w376) -> ()  [unwired: 9 in, 1 out]
              }
              frame Enabled {
              }
            }
          }
          frame #1 {
            n297 = call "test_waypoint-files.vi"() -> ()  [unwired: 12 in]
          }
        }
      }
      event "VLP16 cfg": Value Change {
        n298 = event-data() -> ()  [unwired: 1 in, 1 out]
        n299 = call "fgv_lidar-range_vh.vi"("cmd"=enum16{"read", "write"}."write", "VLP16 cfg"="VLP16 cfg") -> ()  [unwired: 9 in, 1 out]
        n300 = case shown="참" FALSE {
          tunnel: "VLP16 cfg" -> [_ w382]
          frame False {
          }
          frame True {
            n301 = Flatten To XML(anything=w382) -> (xml string=w381:string)
            n302 = call "sub_log_basic.vi"("desc"=w381, "Title"="vlp16 cfg  change") -> ()  [unwired: 9 in, 1 out]
          }
        }
      }
      event "RPLidar cfg": Value Change {
        n303 = event-data() -> ()  [unwired: 1 in, 1 out]
        n304 = call "fgv_rplidar_config.vi"("cmd"=enum16{"read", "write"}."write", "RPLidar cfg"="RPLidar cfg") -> ()  [unwired: 8 in, 2 out]
      }
      event "AGV cfg": Value Change {
        n305 = event-data() -> ()  [unwired: 1 in, 1 out]
        n306 = call "fgv_agv_config.vi"("cmd"=enum16{"read", "write"}."write", "AGV cfg"="AGV cfg") -> ()  [unwired: 8 in, 2 out]
      }
      event "State machine cfg": Value Change {
        n307 = event-data() -> ()  [unwired: 1 in, 1 out]
        n308 = call "fgv_state-machine_config.vi"("cmd"=enum16{"write", "read"}."write", "Angle cfg"="State machine cfg") -> ()  [unwired: 9 in, 1 out]
      }
      event "PID cfg": Value Change {
        n309 = event-data() -> ()  [unwired: 1 in, 1 out]
        n310 = case shown="참" FALSE {
          frame False {
          }
          frame True {
            n311 = call "sub_msgbox.vi"("Reference pid values"=" # Be careful #\n---Ref val--- \np gain: 0.1\nlimit: +- 2000\ndt: 100ms" ("Test title")) -> ()  [unwired: 11 in]
          }
        }
        n312 = call "fgv_pid-config.vi"("cmd"=enum16{"read", "write"}."write", "PID cfg"="PID cfg") -> ()  [unwired: 8 in, 2 out]
      }
      event "speed-steer_global", "decrease ratio": Value Change {
        n313 = event-data() -> ()  [unwired: 1 in, 1 out]
        n314 = call "fgv_agv_speedsteer-common.vi"("cmd"=enum16{"init", "read", "write"}."write", "decrease ratio"="decrease ratio", "speed-steer"="speed-steer_global") -> ()  [unwired: 7 in, 2 out]
      }
      event "waypoint files cfg": Value Change {
        n315 = event-data() -> ()  [unwired: 1 in, 1 out]
        n316 = flat-sequence {
          frame #0 {
            n317 = call "fgv_waypoint_config.vi"("cmd"=enum16{"read", "write"}."write", "waypoint files cfg"="waypoint files cfg") -> ("waypoint files cfg out"=w404:T26)  [unwired: 9 in]
            n318 = call "sub_waypoints_upload.vi"("waypoint group"=w404) -> ("waypt error"=w397:bool, "waypoint all"=w405:cluster{"XY 그래프":cluster{"X":dbl, "Y":dbl}[]}[])  [unwired: 9 in]
            n319 = call "fgv_waypoint_total.vi"("cmd"=enum16{"write", "read"}."write", "waypoint total in"=w405) -> ("waypoint total out"=w403:cluster{"waypt":cluster{"X":dbl, "Y":dbl}[]}[])  [unwired: 9 in]
            n320 = for {
              shift-right: [w421] -> w400
              shift-left: T27 [] -> [w422]
              tunnel: w403 -> [w423] mode=indexing
              n321 = Build Array (concatenate)(w422, w423) -> (w421:cluster{"waypt":cluster{"X":dbl, "Y":dbl}[]}[])
            }
            n322 = call "fgv_stop-point_databuf.vi"("cmd"=enum16{"clear", "write", "read"}."read") -> ("all stop pts out"=w399:cluster{dbl, dbl}[])  [unwired: 10 in]
            n323 = flat-sequence {
              tunnel: w397 -> [w410]
              frame #0 {
                n324 = call "sub_error_data-conversion.vi"("error status"=w410) -> ("error conversion out"=w411:T2)  [unwired: 9 in, 1 out]
                n325 = call "fgv_error-2.vi"("cmd"=enum16{"init", "read", "write"}."read") -> ("Error cluster out"=w414:T42)  [unwired: 9 in, 1 out]
                n326 = Bundle By Name(cluster=w414, "Waypt"=w411) -> (w415:T42)
                n327 = call "fgv_error-2.vi"("cmd"=enum16{"init", "read", "write"}."write", "Error cluster"=w415) -> ()  [unwired: 8 in, 2 out]
              }
            }
            n328 = case shown="거짓" TRUE {
              tunnel: [w416 w419] -> w401
              tunnel: w400 -> [w416 w420]
              tunnel: w399 -> [_ w418]
              frame False {
              }
              frame True {
                n329 = Bundle("all stop pts out"=w418) -> (w417:cluster{"all stop pts out":cluster{dbl, dbl}[]})  [unwired: 1 in]
                n330 = Build Array (concatenate)(w417, w420) -> (w419:T27)
              }
            }
            "Total map cfg" <- w401
          }
        }
      }
      event "config load": Value Change {
        n331 = event-data() -> ()  [unwired: 1 in, 1 out]
        n332 = flat-sequence {
          frame #0 {
            n333 = call "fgv_parameter_save-load.vi"("ctl"=T32."Config Load") -> ()  [unwired: 9 in, 2 out]
          }
          frame #1 {
            n334 = call "sub_control-val_update_from_global.vi"() -> ()  [unwired: 12 in]
          }
        }
      }
      event "config save": Value Change {
        n335 = event-data() -> ()  [unwired: 1 in, 1 out]
        n336 = flat-sequence {
          frame #0 {
            n337 = call "sub_control-val_update_to_global.vi"() -> ()  [unwired: 12 in]
          }
          frame #1 {
            n338 = call "fgv_parameter_save-load.vi"("ctl"=T32."Config Save", "file name"="config_file-name") -> ()  [unwired: 8 in, 2 out]
          }
        }
      }
      event "Checking": Value Change {
        n339 = event-data() -> ()  [unwired: 1 in, 1 out]
        n340 = call "fgv_hw-info.vi"("cmd"=enum16{"write", "read"}."read") -> ("HW info out"=w433:T29)  [unwired: 10 in]
        n341 = Unbundle(w433) -> ("AGV"=w432:T67, "Lidar 1"=w431:T68, "Lidar 2"=w430:T68, "GPS"=w429:T69, "Camera"=w428:T70, "Joystick"=w427:enum16{"none", "joystick"})
        n342 = stacked-sequence {
          tunnel: w432 -> [w438 _ _ _ _ _]
          tunnel: w431 -> [_ w447 _ _ _ _]
          tunnel: w430 -> [_ _ w454 _ _ _]
          tunnel: w429 -> [_ _ _ w455 _ _]
          tunnel: w428 -> [_ _ _ _ w460 _]
          tunnel: w427 -> [_ _ _ _ _ w463]
          frame #0 {
            n343 = case shown="\"Scout\"" w438 {
              frame "ERP42" {
                n344 = call "fgv_erp42_q.vi"("cmd"=enum16{"create", "write", "read", "close"}."write", "data"=enum16{"run", "check", "stop"}."check") -> ()  [unwired: 8 in, 2 out]
              }
              frame "ERP42mini" {
                n345 = call "fgv_erp42mini-232_q.vi"("cmd"=enum16{"create", "write", "read", "close"}."write", "data"=enum16{"run", "check", "stop"}."check") -> ()  [unwired: 8 in, 2 out]
              }
              frame "Scout" {
                n346 = call "fgv_q_agv.vi"("cmd"=enum16{"create", "write", "read", "close"}."write", "data"=enum16{"run", "check", "stop"}."check") -> ()  [unwired: 8 in, 2 out]
              }
              frame "Ycar" {
                n347 = call "fgv_ycar_q.vi"("cmd"=enum16{"create", "write", "read", "close"}."write", "data"=enum16{"run", "check", "stop"}."check") -> ()  [unwired: 8 in, 2 out]
              }
              frame "none", Default {
              }
            }
          }
          frame #1 {
            n348 = case shown="\"none\", 기본" w447 {
              frame "none", Default {
              }
              frame "VLP16" {
                n349 = call "fgv_q_vlp16.vi"("cmd"=enum16{"create", "write", "read", "close"}."write", "data"=enum16{"run", "check", "stop"}."check") -> ()  [unwired: 8 in, 2 out]
              }
              frame "TIM571" {
                n350 = call "fgv_q_tim571.vi"("cmd"=enum16{"create", "write", "read", "close"}."write", "data"=enum16{"run", "check", "stop"}."check") -> ()  [unwired: 8 in, 2 out]
              }
              frame "RPLidar A2", "RPLidar A3" {
                n351 = call "fgv_rplidar_232_q.vi"("cmd"=enum16{"create", "write", "read", "close"}."write", "data"=enum16{"run", "check", "stop"}."check") -> ()  [unwired: 8 in, 2 out]
              }
            }
          }
          frame #2 {
            n352 = case shown="\"VLP16\"" w454 {
              frame "none", Default {
              }
              frame "VLP16" {
              }
            }
          }
          frame #3 {
            n353 = case shown="\"F9P\", \"M8P\"" w455 {
              frame "none", Default {
              }
              frame "F9P", "M8P" {
                n354 = call "fgv_F9P_q.vi"("cmd"=enum16{"create", "write", "read", "close"}."write", "data"=enum16{"run", "check", "stop"}."check") -> ()  [unwired: 8 in, 2 out]
              }
              frame "PwrPak7" {
                n355 = call "fgv_q_PwrPak7.vi"("cmd"=enum16{"create", "write", "read", "close"}."write", "data"=enum16{"run", "check", "stop"}."check") -> ()  [unwired: 8 in, 2 out]
              }
              frame "19X HVS" {
              }
            }
          }
          frame #4 {
            # "Cam"
            n356 = case shown="\"C920\", 기본" w460 {
              frame "none" {
              }
              frame "C920", Default {
                n357 = call "fgv_pc_cam_q.vi"("cmd"=enum16{"create", "write", "read", "close"}."write", "data"=enum16{"run", "check", "stop"}."check") -> ()  [unwired: 8 in, 2 out]
              }
            }
          }
          frame #5 {
            # "joystick"
            n358 = case shown="\"joystick\", 기본" w463 {
              frame "none" {
              }
              frame "joystick", Default {
                n359 = call "fgv_q_joystick.vi"("cmd"=enum16{"create", "write", "read", "close"}."write", "data"=enum16{"run", "check", "stop"}."check") -> ()  [unwired: 8 in, 2 out]
              }
            }
          }
        }
        n360 = property on="start-stop" class="Bool (엄격한)"("DisabledEnum"=T34."Enabled" ("비활성화")) -> ()  [unwired: 2 in, 2 out]
        n361 = call "fgv_status-display.vi"("Mode"=enum16{"Initial", "Update", "Clear"}."Update", "title"="*** HW checking ***" ("String in 1")) -> ()  [unwired: 9 in, 1 out]
      }
      event "LiDAR Display": Mouse Down {
        n362 = event-data() -> ()  [unwired: 1 in, 1 out]
      }
      event "state change": Value Change {
        n363 = event-data() -> ()  [unwired: 1 in, 1 out]
        n364 = call "fgv_system_state.vi"("cmd"=enum16{"init", "read", "write"}."write", "State"="set state value") -> ("State out"=w466:T1)  [unwired: 8 in, 1 out]
        n365 = flat-sequence {
          tunnel: w466 -> [_]
          frame #0 {
            n366 = call "fgv_loop_count.vi"("cmd"=enum16{"init", "read", "write"}."read") -> ()  [unwired: 9 in, 2 out]
          }
        }
      }
      event "Lookahead cfg": Value Change {
        n367 = event-data() -> ()  [unwired: 1 in, 1 out]
        n368 = call "fgv_look-ahead_config.vi"("cmd"=enum16{"read", "write"}."write", "lookahed cfg in"="Lookahead cfg") -> ()  [unwired: 9 in, 1 out]
      }
      event "start-stop": Value Change {
        n369 = event-data() -> ()  [unwired: 1 in, 1 out]
        n370 = case shown="참" "start-stop" {
          frame False {
            n371 = call "fgv_local-stop_agv.vi"("cmd"=enum16{"ini", "read", "stop"}."stop") -> ()  [unwired: 10 in, 1 out]
            n372 = property on="Checking" class="Bool"("DisabledEnum"=T34."Enabled" ("비활성화")) -> ()  [unwired: 2 in, 2 out]
            n373 = call "sub_system_pause-condition.vi"("cmd"=enum16{"pause", "go", "read"}."pause") -> ()  [unwired: 10 in, 1 out]
            n374 = disable-structure shown="비활성화" {
              frame Disabled {
                n375 = property on="start-stop" class="Bool (엄격한)" props=["DisabledEnum"]() -> ()  [unwired: 3 in, 2 out]
              }
              frame Enabled {
              }
            }
            n376 = call "fgv_status-display.vi"("Mode"=enum16{"Initial", "Update", "Clear"}."Update", "detail"="----Stop----", "title"="" ("String in 1")) -> ()  [unwired: 8 in, 1 out]
          }
          frame True {
            n377 = flat-sequence {
              frame #0 {
                n378 = call "fgv_local-stop_agv.vi"("cmd"=enum16{"ini", "read", "stop"}."ini") -> ()  [unwired: 10 in, 1 out]
                n379 = call "sub_system_pause-condition.vi"("cmd"=enum16{"pause", "go", "read"}."go") -> ()  [unwired: 10 in, 1 out]
              }
              frame #1 {
                n380 = call "fgv_hw-info.vi"("cmd"=enum16{"write", "read"}."read") -> ("HW info out"=w488:T29)  [unwired: 10 in]
                n381 = Unbundle(w488) -> ("AGV"=w487:T67, "Lidar 1"=w486:T68, "Lidar 2"=w485:T68, "GPS"=w484:T69, "Camera"=w483:T70, "Joystick"=w481:enum16{"none", "joystick"})
                n382 = stacked-sequence {
                  tunnel: w487 -> [w489 _ _ _ _ _]
                  tunnel: w486 -> [_ w498 _ _ _ _]
                  tunnel: w485 -> [_ _ w505 _ _ _]
                  tunnel: w484 -> [_ _ _ w506 _ _]
                  tunnel: w483 -> [_ _ _ _ w513 _]
                  tunnel: w481 -> [_ _ _ _ _ w514]
                  frame #0 {
                    n383 = case shown="\"ERP42\"" w489 {
                      frame "ERP42" {
                        n384 = call "fgv_erp42_q.vi"("cmd"=enum16{"create", "write", "read", "close"}."write", "data"=enum16{"run", "check", "stop"}."run") -> ()  [unwired: 8 in, 2 out]
                      }
                      frame "ERP42mini" {
                        n385 = call "fgv_erp42mini-232_q.vi"("cmd"=enum16{"create", "write", "read", "close"}."write", "data"=enum16{"run", "check", "stop"}."run") -> ()  [unwired: 8 in, 2 out]
                      }
                      frame "Scout" {
                        n386 = call "fgv_q_agv.vi"("cmd"=enum16{"create", "write", "read", "close"}."write", "data"=enum16{"run", "check", "stop"}."run") -> ()  [unwired: 8 in, 2 out]
                      }
                      frame "Ycar" {
                        n387 = call "fgv_ycar_q.vi"("cmd"=enum16{"create", "write", "read", "close"}."write", "data"=enum16{"run", "check", "stop"}."run") -> ()  [unwired: 8 in, 2 out]
                      }
                      frame "none", Default {
                      }
                    }
                  }
                  frame #1 {
                    n388 = case shown="\"TIM571\"" w498 {
                      frame "none", Default {
                      }
                      frame "VLP16" {
                        n389 = call "fgv_q_vlp16.vi"("cmd"=enum16{"create", "write", "read", "close"}."write", "data"=enum16{"run", "check", "stop"}."run") -> ()  [unwired: 8 in, 2 out]
                      }
                      frame "TIM571" {
                        n390 = call "fgv_q_tim571.vi"("cmd"=enum16{"create", "write", "read", "close"}."write", "data"=enum16{"run", "check", "stop"}."run") -> ()  [unwired: 8 in, 2 out]
                      }
                      frame "RPLidar A2", "RPLidar A3" {
                        n391 = call "fgv_rplidar_232_q.vi"("cmd"=enum16{"create", "write", "read", "close"}."write", "data"=enum16{"run", "check", "stop"}."run") -> ()  [unwired: 8 in, 2 out]
                      }
                    }
                  }
                  frame #2 {
                    n392 = case shown="\"TIM571\"" w505 {
                      frame "none", Default {
                      }
                      frame "VLP16" {
                      }
                      frame "TIM571" {
                      }
                      frame "RPLidar A2" {
                      }
                      frame "RPLidar A3" {
                      }
                    }
                  }
                  frame #3 {
                    n393 = case shown="\"none\", 기본" w506 {
                      frame "none", Default {
                      }
                      frame "F9P", "M8P" {
                        n394 = call "fgv_F9P_q.vi"("cmd"=enum16{"create", "write", "read", "close"}."write", "data"=enum16{"run", "check", "stop"}."run") -> ()  [unwired: 8 in, 2 out]
                      }
                      frame "PwrPak7" {
                        n395 = call "fgv_q_PwrPak7.vi"("cmd"=enum16{"create", "write", "read", "close"}."write", "data"=enum16{"run", "check", "stop"}."run") -> ()  [unwired: 8 in, 2 out]
                      }
                      frame "19X HVS" {
                      }
                    }
                  }
                  frame #4 {
                    n396 = case shown="\"C920\"" w513 {
                      frame "none", Default {
                      }
                      frame "C920" {
                      }
                    }
                    n397 = call "fgv_pc_cam_q.vi"("cmd"=enum16{"create", "write", "read", "close"}."write", "data"=enum16{"run", "check", "stop"}."run") -> ()  [unwired: 8 in, 2 out]
                  }
                  frame #5 {
                    n398 = case shown="\"joystick\"" w514 {
                      frame "none", Default {
                      }
                      frame "joystick" {
                        n399 = call "fgv_q_joystick.vi"("cmd"=enum16{"create", "write", "read", "close"}."write", "data"=enum16{"run", "check", "stop"}."run") -> ()  [unwired: 8 in, 2 out]
                      }
                    }
                  }
                }
              }
              frame #2 {
                n400 = property on="pause-resume" class="Bool (엄격한)"("DisabledEnum"=T34."Enabled" ("비활성화")) -> ()  [unwired: 2 in, 2 out]
                n401 = property on="Checking" class="Bool"("DisabledEnum"=T34."Disabled and Grayed Out" ("비활성화")) -> ()  [unwired: 2 in, 2 out]
                n402 = call "fgv_status-display.vi"("Mode"=enum16{"Initial", "Update", "Clear"}."Update", "detail"="----Start----", "title"="" ("String in 1")) -> ()  [unwired: 8 in, 1 out]
              }
            }
          }
        }
      }
      event "Joystick\ncontrol": Value Change {
        n403 = event-data() -> ()  [unwired: 1 in, 1 out]
        n404 = call "fgv_error-2.vi"("cmd"=enum16{"init", "read", "write"}."read") -> ("Error cluster out"=w527:T42)  [unwired: 9 in, 1 out]
        n405 = Unbundle By Name(w527) -> ("Joystick"=w525:T2)
        n406 = Equal?(x=w525, y=T2 2) -> (x = y?=w523:bool)
        n407 = And(x=w523, y="Joystick\ncontrol") -> (x .and. y?=w522:bool)
        n408 = case shown="거짓" w522 {
          frame False {
            n409 = call "sub_msgbox.vi"("Reference pid values"=" joystick is not ready" ("Test title")) -> ()  [unwired: 11 in]
            n410 = call "fgv_joystick-info.vi"("init"=enum16{"enable", "init", "read", "write"}."init") -> ()  [unwired: 7 in, 4 out]
          }
          frame True {
            n411 = call "fgv_joystick-info.vi"("init"=enum16{"enable", "init", "read", "write"}."enable") -> ()  [unwired: 7 in, 4 out]
          }
        }
      }
      event "Record waypoint": Value Change {
        n412 = event-data() -> ()  [unwired: 1 in, 1 out]
      }
      event "GPS cfg": Value Change {
        n413 = event-data() -> ()  [unwired: 1 in, 1 out]
        n414 = call "fgv_gps_config.vi"("cmd"=enum16{"read", "write"}."write", "cfg"="GPS cfg") -> ()  [unwired: 8 in, 2 out]
      }
      event Value Change {
        n415 = event-data() -> ()  [unwired: 1 in, 1 out]
        n416 = call "fgv_joystick_config.vi"("cmd"=cmd_common."write", "Joystick cfg"="Joystick cfg") -> ()  [unwired: 8 in, 2 out]
      }
      event "Speed": Value Change {
        n417 = event-data() -> ()  [unwired: 1 in, 1 out]
        n418 = flat-sequence {
          tunnel: "Speed" -> [w537]
          frame #0 {
            n419 = call "fgv_erp42_opval.vi"("cmd"=enum16{"read", "write", "ini"}."read") -> ("data_out"=w541:T66)  [unwired: 10 in]
            n420 = Bundle By Name(cluster=w541, "Drive_value.Speed"=w537) -> (w540:T66)
            n421 = call "fgv_erp42_opval.vi"("cmd"=enum16{"read", "write", "ini"}."write", "data_in"=w540) -> ()  [unwired: 9 in, 1 out]
          }
        }
      }
      event Value Change {
        n422 = event-data() -> ()  [unwired: 1 in, 1 out]
        n423 = call "fgv_hw-info.vi"("cmd"=enum16{"write", "read"}."write", "HW info"="HW info") -> ()  [unwired: 9 in, 1 out]
      }
      event "Obstacle limit cfg": Value Change {
        n424 = event-data() -> ()  [unwired: 1 in, 1 out]
        n425 = call "fgv_obstacle_data.vi"("cmd"=obstacle_info."write limit", "limit in"="Obstacle limit cfg") -> ()  [unwired: 6 in, 4 out]
      }
      event "close": Value Change {
        n426 = event-data() -> ()  [unwired: 1 in, 1 out]
        n427 = flat-sequence {
          tunnel: [w549] -> w546
          tunnel: [w566] -> w547
          tunnel: w546 -> [w566]
          frame #0 {
            n428 = case shown="참" TRUE {
              tunnel: [FALSE ("stop status") w558] -> w549
              frame False {
              }
              frame True {
                n429 = call "fgv_q_vlp16.vi"("cmd"=enum16{"create", "write", "read", "close"}."close") -> ()  [unwired: 9 in, 2 out]
                n430 = call "fgv_erp42_q.vi"("cmd"=enum16{"create", "write", "read", "close"}."close") -> ()  [unwired: 9 in, 2 out]
                n431 = call "fgv_rplidar_232_q.vi"("cmd"=enum16{"create", "write", "read", "close"}."close") -> ()  [unwired: 9 in, 2 out]
                n432 = call "fgv_q_PwrPak7.vi"("cmd"=enum16{"create", "write", "read", "close"}."close") -> ()  [unwired: 9 in, 2 out]
                n433 = call "fgv_F9P_q.vi"("cmd"=enum16{"create", "write", "read", "close"}."close") -> ()  [unwired: 9 in, 2 out]
                n434 = call "fgv_erp42mini-232_q.vi"("cmd"=enum16{"create", "write", "read", "close"}."close") -> ()  [unwired: 9 in, 2 out]
                n435 = call "fgv_q_tim571.vi"("cmd"=enum16{"create", "write", "read", "close"}."close") -> ()  [unwired: 9 in, 2 out]
                n436 = call "fgv_pc_cam_q.vi"("cmd"=enum16{"create", "write", "read", "close"}."close") -> ()  [unwired: 9 in, 2 out]
                n437 = call "fgv_ycar_q.vi"("cmd"=enum16{"create", "write", "read", "close"}."close") -> ()  [unwired: 9 in, 2 out]
                n438 = call "fgv_logbuff_q.vi"("cmd"=log_buffq."close") -> ()  [unwired: 9 in, 2 out]
                n439 = call "fgv_q_agv.vi"("cmd"=enum16{"create", "write", "read", "close"}."close") -> ()  [unwired: 9 in, 2 out]
                n440 = call "fgv_q_joystick.vi"("cmd"=enum16{"create", "write", "read", "close"}."close") -> ()  [unwired: 9 in, 2 out]
                n441 = call "fgv_global-stop.vi"("cmd"=enum16{"init", "stop", "read"}."stop") -> ("val_out"=w558:bool)  [unwired: 10 in]
              }
            }
          }
          frame #1 {
            n442 = local write "close"(FALSE ("close")) -> ()
          }
        }
      }
      event "pause-resume": Value Change {
        n443 = event-data() -> ()  [unwired: 1 in, 1 out]
        n444 = case shown="거짓" "pause-resume" {
          frame False {
            n445 = call "sub_system_pause-condition.vi"("cmd"=enum16{"pause", "go", "read"}."go") -> ()  [unwired: 10 in, 1 out]
            n446 = call "fgv_status-display.vi"("Mode"=enum16{"Initial", "Update", "Clear"}."Update", "title"="----Go----" ("String in 1")) -> ()  [unwired: 9 in, 1 out]
          }
          frame True {
            n447 = call "sub_system_pause-condition.vi"("cmd"=enum16{"pause", "go", "read"}."pause") -> ()  [unwired: 10 in, 1 out]
            n448 = call "fgv_status-display.vi"("Mode"=enum16{"Initial", "Update", "Clear"}."Update", "title"="----Pause----" ("String in 1")) -> ()  [unwired: 9 in, 1 out]
          }
        }
      }
      event "TIM571 cfg": Value Change {
        n449 = event-data() -> ()  [unwired: 1 in, 1 out]
        n450 = call "fgv_tim571_setting.vi"("cmd"=enum16{"write", "read"}."write", "tim571_setting-data_in"="TIM571 cfg") -> ()  [unwired: 9 in, 1 out]
      }
    }
  }
  n451 = while {
    tunnel: w2 -> [_]
    stop <- w576 stop-if-true
    n452 = call "fgv_error-2.vi"("cmd"=enum16{"init", "read", "write"}."read") -> ("Error cluster out"=w579:T42)  [unwired: 9 in, 1 out]
    n453 = Unbundle By Name(w579) -> ("GNSS"=w578:T2)
    n454 = case shown="0" w578 {
      frame 0 {
        n455 = Wait (ms)(milliseconds to wait=u32 1000 ("대기 시간 (ms)")) -> ()  [unwired: 1 out]
      }
      frame 2, Default {
        n456 = call "fgv_agv_position.vi"("cmd"=enum16{"write", "read"}."read") -> ("latlong out"=w585:cluster{dbl, dbl})  [unwired: 8 in, 2 out]
        "latlong out" <- w585
        n457 = local read "PinDropMrkr"() -> (w586:T12)
        n458 = call "fgv_gmap_core.vi"("cmd"=gmap_fgv-cmd."clear marker") -> ("error out"=w588:errorcluster)  [unwired: 7 in, 3 out]
        n459 = Cluster To Array(cluster=w585) -> (array=w587:dbl[])
        n460 = Bundle("latlong out"=w587, "PinDropMrkr"=w586) -> (w582:T71)  [unwired: 1 in]
        n461 = flat-sequence {
          tunnel: w588 -> [w592]
          tunnel: w582 -> [w593]
          tunnel: [w593] -> w590
          tunnel: [w592] -> w589
          tunnel: w590 -> [w596]
          tunnel: w589 -> [w595]
          frame #0 {
            n462 = Wait (ms)(milliseconds to wait=u32 20) -> ()  [unwired: 1 out]
          }
          frame #1 {
            n463 = call "fgv_gmap_core.vi"("cmd"=gmap_fgv-cmd."add marker", "error in"=w595, "marker_info"=w596) -> ()  [unwired: 5 in, 4 out]
            n464 = Wait (ms)(milliseconds to wait=u32 1000) -> ()  [unwired: 1 out]
          }
        }
      }
    }
    n465 = call "fgv_global-stop.vi"("cmd"=enum16{"init", "stop", "read"}."read") -> ("val_out"=w576:bool)  [unwired: 10 in]
  }
  n466 = disable-structure shown="비활성화" {
    disable-tunnel: w1 -> [w598 _]
    frame Disabled {
      n467 = call "sub_main_pwrpak7.vi"("error in"=w598) -> ()  [unwired: 10 in, 1 out]
      n468 = call "sub_main_agv.vi"("error in"=w598) -> ()  [unwired: 10 in, 1 out]
    }
    frame Enabled {
    }
  }
  n469 = Merge Errors(w46, w50, w49, w48, w47, w40, w39, w38) -> (w37:errorcluster)
  n470 = call "sub_cam_main.vi"("error in"=w1) -> ("error out"=w45:errorcluster)  [unwired: 10 in]
  n471 = call "sub_main_vision.vi"("error in"=w1) -> ("error out"=w44:errorcluster)  [unwired: 10 in]
  n472 = call "sub_main_timer.vi"("error in"=w1) -> ("error out"=w43:errorcluster)  [unwired: 10 in]
  n473 = call "sub_main_data-process.vi"("error in"=w1) -> ("error out"=w42:errorcluster)  [unwired: 10 in]
  n474 = call "sub_main_pid.vi"("error in"=w1) -> ("error out"=w33:errorcluster)  [unwired: 10 in]
  n475 = call "sub_main_speed-control.vi"("error in"=w1) -> ("error out"=w34:errorcluster)  [unwired: 10 in]
  n476 = call "sub_main_state.vi"("error in"=w1) -> ("error out"=w35:errorcluster)  [unwired: 10 in]
  n477 = call "sub_main_appcomm.vi"("error in"=w1) -> ("error out"=w36:errorcluster)  [unwired: 10 in]
  n478 = call "sub_main_joystick.vi"("error in"=w1) -> ("error out"=w31:errorcluster)  [unwired: 10 in]
  n479 = Merge Errors(w45, w44, w43, w42, w33, w34, w35, w36, w31) -> (w32:errorcluster)
  n480 = flat-sequence {
    tunnel: w1 -> [_]
    frame #0 {
      # "wpt"
    }
  }
  n481 = flat-sequence {
    tunnel: w1 -> [_]
    frame #0 {
      # "Gmap\n.net"
    }
  }
  n482 = call "sub_rplidar_main.vi"("error in"=w1) -> ("error out"=w29:errorcluster)  [unwired: 10 in]
  n483 = call "sub_main_ycar.vi"("error in"=w1) -> ("error out"=w28:errorcluster)  [unwired: 10 in]
  n484 = Merge Errors(w29, w28) -> (w30:errorcluster)
  n485 = flat-sequence {
    tunnel: w52 -> [_]
    tunnel: [w599] -> w51
    frame #0 {
      n486 = call "fgv_status-display.vi"("Mode"=enum16{"Initial", "Update", "Clear"}."Update", "title"="Producer fihish" ("String in 1")) -> ("error out"=w599:errorcluster)  [unwired: 9 in]
    }
  }
  n487 = Merge Errors(w30, w32, w37) -> (w41:errorcluster)
  n488 = flat-sequence {
    tunnel: w51 -> [_]
    tunnel: w41 -> [_]
    frame #0 {
      n489 = call "sub_update-parameters-to-global for save.vi"() -> ()  [unwired: 12 in]
    }
    frame #1 {
      n490 = call "sub_control-val_update_to_global.vi"() -> ()  [unwired: 12 in]
    }
    frame #2 {
      n491 = call "fgv_parameter_save-load.vi"("ctl"=T32."LastRUN Save") -> ()  [unwired: 9 in, 2 out]
      n492 = call "fgv_lidars-img.vi"("cmd"=enum16{"create", "read", "close"}."close") -> ()  [unwired: 10 in, 1 out]
      n493 = call "sub_register-event-callback.vi"("cmd"=enum16{"register", "close"}."close") -> ("error out"=w602:errorcluster)  [unwired: 10 in]
      n494 = call "fgv_gmap_core.vi"("cmd"=gmap_fgv-cmd."close", "error in"=w602) -> ()  [unwired: 6 in, 4 out]
      n495 = call "fgv_status-display.vi"("Mode"=enum16{"Initial", "Update", "Clear"}."Update", "title"="Shut down" ("String in 1")) -> ()  [unwired: 9 in, 1 out]
    }
    frame #3 {
      n496 = disable-structure shown="Disabled" {
        frame Disabled {
          n497 = Array To Spreadsheet String(array=string[] ["GNSS Week", "GNSS sec", "Pos Type_GNSS", "INS_Status", "Pos Type_INS", "Lat", "Lon", "Height", "Heading", "North Vel", "East Vel", "Up Vel", "Roll", "Pitch", "Azimuth", "Lat σ ", "Lon σ", "Height σ", "North Vel σ", "East Vel σ", "Up Vel σ", "Roll σ", "Pitch σ", "Azimuth σ", "Heading σ"], 3:"" ("포맷 문자열")) -> (spreadsheet string=w609:string)  [unwired: 1 in]
          n498 = call "sub_log_scout.vi"("str"=w609) -> ()  [unwired: 10 in, 1 out]
        }
        frame Enabled {
        }
      }
    }
    frame #4 {
      n499 = case shown="거짓" FALSE {
        frame False {
        }
        frame True {
          n500 = call "IMAQ Dispose"("All Images? (No)"=TRUE) -> ()  [unwired: 5 in, 1 out]
        }
      }
      n501 = local write "close"(FALSE ("stop")) -> ()
    }
  }
